vi "ME_acquire_18_DeltaForce_Daq_SteppingMode.vi"() -> ()   [LabVIEW 2015]
doc: "Use this template to build a producer/consumer design pattern. Use this template when you need to execute a process, such as data analysis, when a data source, such as a triggered acquisition, produces data at an uneven rate and you need to execute the process when the data becomes available."
uses:
  oxford_driver/Oxford Drivers/BUSGEN.LLB/OxfordAddress.ctl
  <vilib>/express/express arith-compare/Formula/XNode/ExpressFormulaBlockNode.xnode
  Mode.ctl
  <vilib>/Utility/file.llb/Write Delimited Spreadsheet (DBL).vi
  <vilib>/Analysis/NI_AALBase.lvlib
  <vilib>/Analysis/baseanly.llb/Mean (DBL).vi
  <vilib>/DAQmx/configure/timing.llb/DAQmx Timing (Sample Clock).vi
  <vilib>/DAQmx/create/channels.llb/DAQmx Create Channel (AI-Voltage-Basic).vi
  <vilib>/DAQmx/read.llb/DAQmx Read (Analog 1D DBL 1Chan NSamp).vi
panel:
  out "element":dbl
  out "TimeUp":bool
  out "meanPolarization":dbl format="%0.2f"
  out "Polarization array":dbl[](array[numeric])
  in  "First Offset?":bool
  out "Last2":dbl
  out "Actual2":dbl
  out "Up/Down":bool
  out "T array":dbl[](array[numeric])
  out "Averaged I(T)":dbl[][](array[numeric])
  in  "Averaged P(T)":dbl[][](array[numeric])
  out "remaining elements 2":T1(array[cluster])
  out "Actual mean":dbl format="%0.6f"
  in  "Averaged dt":dbl[][](array[numeric])
  in  "Averaged P(B)":dbl[][](array[numeric])
  out "LockInR":dbl
  out "deltaUaux":dbl
  out "Actual Voltage (V)":dbl caption="Actual AuxV" step=0.1
  in  "Stop":bool
  out "SaveSweep":bool=TRUE
  out "Measurement File_dn":path
  out "Measurement File_up":path
  out "Measurement File_average":path
  out "Actual Polarization":dbl
  in  "Reset IB?":bool
  in  "First?":bool
  in  "Save Period":dbl=1.0
  out "Averaged I(B)":dbl[][](array[numeric])
  out "P(uC/mm^2)":dbl[](array[numeric])
  in  "Sweep":bool
  out "Offset array":dbl[](array[numeric])
  in  "stop 2":bool
  in  "dB":dbl=0.005
  out "appended array":dbl[][](array[numeric])
  out "Actual B Field (T)":dbl
  out "Actual Temperature (K)":dbl
  out "Actual Current (pA)":dbl
  in  "Tab Control":T2(tab)
  in  "dt (K)":dbl=0.1
  in  "Max temperature (K)":dbl=20.0
  in  "Min Temperature (K)":dbl=4.5
  out "P(T)":cluster{dbl[], dbl[]}[](graph)
  out "I(T)":cluster{dbl[], dbl[]}[](graph)
  in  "Set temperature (K)":dbl=4.5
  in  "Temp Ramping Rate (K/min)":dbl=10.0
  in  "Heater Range":enum16{"Off", "Low", "Medium", "High"}(ring)
  in  "Heater On/Off":bool
  out "Setpoint Temperature (K)":dbl
  out "I(T) /Averaged/":cluster{"B array":dbl[], dbl[]}[](graph)
  out "P(T) /Averaged/":cluster{"B array":dbl[], dbl[]}[](graph)
  in  "Stabilization Time (s)":dbl
  out "I(B) 3":cluster{dbl[], dbl[]}[](graph)
  out "I(B) /Averaged/":cluster{"B array":dbl[], dbl[]}[](graph)
  out "P(B) /Averaged/":cluster{"B array":dbl[], dbl[]}[](graph)
  out "P(B)":cluster{"yi":dbl[], dbl[]}(graph)
  in  "Set Field (T)":dbl
  in  "Go to Set":bool
  in  "Sweep Rate (T/min)":dbl=2.0 format="%.6f"
  in  "Field To Zero":bool
  out "Target Field":dbl
  in  "Min Field (T)":dbl
  in  "Max Field (T)":dbl=0.15
  in  "Threshold B (T)":dbl
  in  "ReOffset":bool
  in  "Window (s)":dbl
  in  "Field Step (T)":dbl
  in  "Stepping Mode":bool
  out "Ready2Step":bool
  in  "Dwell Time (s)":dbl
  out "B(t)":dbl(graph)
  out "I(t)":dbl(graph)
  out "P(t)":dbl(graph)
  in  "Max count array":i32[](array[numeric])=[2]
  in  "Magnetic Field array (T)":dbl[](array[numeric])=[0.025, 0.05, 0.075, 0.1, 0.125, 0.15, 0.175, 0.2, 0.225, 0.25, 0.275, 0.3]
  in  "T Sweep Rate Array":dbl[](array[numeric])=[10.0, 20.0]
  in  "secs to wait":dbl=180.0
  out "Wait (s)":dbl
  in  "Directory":string
  out "Finished":bool=TRUE
  out "Step Rate":bool
  out "New":bool=TRUE
  in  "Temperature Array":dbl[](array[numeric])=[4.5, 5.0, 6.0, 7.0, 8.0, 9.0, 10.0, 11.0, 12.0]
  in  "Sweep Rate Array":dbl[](array[numeric])=[2.0, 1.0, 0.5, 0.1, 0.05, 9.0, 10.0, 11.0, 12.0]
  in  "Record ALL":bool
  in  "Max Countl":i32
  out "i":i32
  out "j":i32
  out "Step Temp":bool
  in  "FileName":string
  in  "Measure Noise":bool
  in  "Cycles":i32
  in  "maximum value":dbl=10.0 format="%0.2f"
  in  "minimum value":dbl=-10.0 format="%0.2f"
  in  "physical channels":tag="Dev1/ai1"
  out "PSD (pA/Hz^1/2) Peaks Removed":cluster{"f0":dbl, "df":dbl, "magnitude":dbl[]}(graph)
  out "PSD (pA/Hz^1/2)":cluster{"f0":dbl, "df":dbl, "magnitude":dbl[]}(graph)
  out "Current (pA) Filtered":waveform(dbl)(graph)
  out "Current (pA)":dbl[](graph)
  in  "Samples per channel":i32=1000
  in  "Rate":dbl=1000.0 format="%0.2f"
  in  "Cut-Off Frequency":dbl=100.0 caption="Lower Cut-Off"
  in  "Filter On":bool
  in  "Count":i32=60
  in  "Keithley (IV conv) averaging":i32=10
  in  "Lock_in_Amplifier":refnum<visa-resource-name>="GPIB0::5::INSTR"
  out "Dc offset":dbl
  in  "Calibrate":bool
  in  "IV converter":refnum<visa-resource-name>="GPIB0::20::INSTR"
  in  "Magnetic Field":refnum<visa-resource-name>="GPIB0::21::INSTR"
  out "Time Lag":dbl=0.0500025749206543
  in  "Lake Shore":refnum<visa-resource-name>="GPIB0::11::INSTR"
  in  "Temp Refresh (s)":dbl=0.1
  in  "Sampling rate (Hz)":dbl=10.0
  in  "Gain (V/A)":dbl=1000000000.0
  in  "Sample area (mm^2)":dbl=1.0
  out "B_V":cluster{dbl[], "Best Linear Fit":dbl[]}[](graph)=[{[-0.00769241141, -0.00768011662, -0.0029394633, 0.00271952438, 0.00937200583, 0.0154641889, 0.0217080684, 0.0281692221, 0.0344763397, 0.0407091529, 0.0473661569, 0.0541476438, 0.0611164384, 0.0676637725, 0.073937413, 0.0801511723, 0.0863882257, 0.0933787866, 0.0997676928, 0.106163316, 0.113953626, 0.118979018, 0.126030157, 0.132855724, 0.13883398, 0.14631074, 0.153030676, 0.159156864, 0.165801088, 0.17248087, 0.178555009, 0.185285367, 0.192834407, 0.198751051, 0.205413053, 0.212847389, 0.219477697, 0.225574642, 0.232225854, 0.239015189, 0.245675966, 0.252411162, 0.258453848, 0.265211852, 0.271251534, 0.277801221, 0.284008329, 0.291402813, 0.297970768, 0.304082546, 0.310761405, 0.317366634, 0.323522001, 0.330123184, 0.336841279, 0.343557963, 0.349608435, 0.356238003, 0.363590921, 0.370338319, 0.376962983], "Best Linear Fit"=[0.0, 0.0015, 0.0035, 0.0056, 0.0076, 0.0096, 0.0116, 0.0136, 0.0156, 0.0177, 0.0197, 0.0219, 0.0239, 0.0259, 0.0279, 0.0299, 0.032, 0.034, 0.036, 0.038, 0.04, 0.042, 0.0441, 0.046, 0.048, 0.05, 0.052, 0.054, 0.056, 0.058, 0.06, 0.0621, 0.0643, 0.0663, 0.0684, 0.0704, 0.0725, 0.0745, 0.0765, 0.0787, 0.0807, 0.0827, 0.0847, 0.0868, 0.0888, 0.0908, 0.0928, 0.0948, 0.0968, 0.0988, 0.1008, 0.1028, 0.1048, 0.1069, 0.1091, 0.1111, 0.1131, 0.1152, 0.1173, 0.1193, 0.1213]}, {[-0.00769241141, -0.00768011662, -0.0029394633, 0.00271952438, 0.00937200583, 0.0154641889, 0.0217080684, 0.0281692221, 0.0344763397, 0.0407091529, 0.0473661569, 0.0541476438, 0.0611164384, 0.0676637725, 0.073937413, 0.0801511723, 0.0863882257, 0.0933787866, 0.0997676928, 0.106163316, 0.113953626, 0.118979018, 0.126030157, 0.132855724, 0.13883398, 0.14631074, 0.153030676, 0.159156864, 0.165801088, 0.17248087, 0.178555009, 0.185285367, 0.192834407, 0.198751051, 0.205413053, 0.212847389, 0.219477697, 0.225574642, 0.232225854, 0.239015189, 0.245675966, 0.252411162, 0.258453848, 0.265211852, 0.271251534, 0.277801221, 0.284008329, 0.291402813, 0.297970768, 0.304082546, 0.310761405, 0.317366634, 0.323522001, 0.330123184, 0.336841279, 0.343557963, 0.349608435, 0.356238003, 0.363590921, 0.370338319, 0.376962983], "Best Linear Fit"=[0.002353460844818253, 0.002357267374965663, 0.003824997997530172, 0.005577049655813272, 0.007636692089275871, 0.009522863265806463, 0.01145600043639222, 0.013456406815525209, 0.015409122826751182, 0.01733883381400479, 0.019399876452181594, 0.021499459635718428, 0.023657034245452215, 0.025684122519169482, 0.027626473848249778, 0.02955028565017564, 0.03148130942513291, 0.03364562299316916, 0.03562366117513693, 0.037603778974812686, 0.040015698972850115, 0.04157158615356273, 0.04375465501257369, 0.04586788562152819, 0.0477187843918964, 0.050033627699098075, 0.05211415440778254, 0.05401085368533849, 0.056067939569859164, 0.05813603439385595, 0.06001661903361471, 0.06210037244704129, 0.06443759401357516, 0.0662694173922171, 0.06833200743687069, 0.07063371605572277, 0.07268649347515121, 0.0745741389696738, 0.07663338837489471, 0.07873540137051047, 0.08079761214887074, 0.08288286343195213, 0.08475371006132383, 0.08684602281837933, 0.08871593939391825, 0.09074375613756333, 0.09266550866283872, 0.09495487889775463, 0.09698835150804998, 0.09888058937557581, 0.10094839843403076, 0.10299341126621803, 0.10489914451207855, 0.10694290468187984, 0.10902286140750632, 0.11110238128028392, 0.11297563849525552, 0.11502818680688229, 0.1173046879946565, 0.11939371707962458, 0.12144474708765744]}]
  out "V_I":cluster{dbl[], "Best Linear Fit":dbl[]}[](graph)=[{[0.0, 0.012, 0.026, 0.04, 0.054, 0.068, 0.081, 0.096, 0.11, 0.124, 0.138, 0.153, 0.167, 0.18, 0.195, 0.208, 0.223, 0.236, 0.251, 0.265, 0.279, 0.292, 0.306, 0.32, 0.334, 0.348, 0.362, 0.375, 0.389, 0.403, 0.417, 0.432, 0.446, 0.46, 0.475, 0.489, 0.504, 0.517, 0.531, 0.546, 0.56, 0.574, 0.588, 0.602, 0.616, 0.63, 0.644, 0.658, 0.672, 0.685, 0.699, 0.713, 0.727, 0.742, 0.755, 0.77, 0.784, 0.799, 0.814, 0.827, 0.841], "Best Linear Fit"=[-0.00769241141, -0.00768011662, -0.0029394633, 0.00271952438, 0.00937200583, 0.0154641889, 0.0217080684, 0.0281692221, 0.0344763397, 0.0407091529, 0.0473661569, 0.0541476438, 0.0611164384, 0.0676637725, 0.073937413, 0.0801511723, 0.0863882257, 0.0933787866, 0.0997676928, 0.106163316, 0.113953626, 0.118979018, 0.126030157, 0.132855724, 0.13883398, 0.14631074, 0.153030676, 0.159156864, 0.165801088, 0.17248087, 0.178555009, 0.185285367, 0.192834407, 0.198751051, 0.205413053, 0.212847389, 0.219477697, 0.225574642, 0.232225854, 0.239015189, 0.245675966, 0.252411162, 0.258453848, 0.265211852, 0.271251534, 0.277801221, 0.284008329, 0.291402813, 0.297970768, 0.304082546, 0.310761405, 0.317366634, 0.323522001, 0.330123184, 0.336841279, 0.343557963, 0.349608435, 0.356238003, 0.363590921, 0.370338319, 0.376962983]}, {[0.0, 0.012, 0.026, 0.04, 0.054, 0.068, 0.081, 0.096, 0.11, 0.124, 0.138, 0.153, 0.167, 0.18, 0.195, 0.208, 0.223, 0.236, 0.251, 0.265, 0.279, 0.292, 0.306, 0.32, 0.334, 0.348, 0.362, 0.375, 0.389, 0.403, 0.417, 0.432, 0.446, 0.46, 0.475, 0.489, 0.504, 0.517, 0.531, 0.546, 0.56, 0.574, 0.588, 0.602, 0.616, 0.63, 0.644, 0.658, 0.672, 0.685, 0.699, 0.713, 0.727, 0.742, 0.755, 0.77, 0.784, 0.799, 0.814, 0.827, 0.841], "Best Linear Fit"=[-0.015941127780698654, -0.010342478990544012, -0.0038107220686969304, 0.0027210348531501527, 0.009252791774997235, 0.01578454869684432, 0.02184975155284518, 0.028848062540538483, 0.03537981946238557, 0.041911576384232645, 0.048443333306079736, 0.05544164429377303, 0.061973401215620116, 0.06803860407162098, 0.07503691505931429, 0.08110211791531513, 0.08810042890300844, 0.0941656317590093, 0.10116394274670261, 0.1076956996685497, 0.11422745659039678, 0.12029265944639762, 0.1268244163682447, 0.1333561732900918, 0.13988793021193888, 0.14641968713378595, 0.15295144405563305, 0.15901664691163392, 0.165548403833481, 0.1720801607553281, 0.17861191767717516, 0.18561022866486845, 0.19214198558671555, 0.19867374250856262, 0.20567205349625592, 0.212203810418103, 0.2192021214057963, 0.22526732426179719, 0.23179908118364426, 0.23879739217133758, 0.24532914909318465, 0.2518609060150317, 0.2583926629368788, 0.2649244198587259, 0.271456176780573, 0.27798793370242003, 0.28451969062426713, 0.29105144754611423, 0.2975832044679613, 0.3036484073239622, 0.31018016424580924, 0.3167119211676563, 0.3232436780895034, 0.3302419890771967, 0.3363071919331976, 0.3433055029208909, 0.34983725984273795, 0.35683557083043127, 0.36383388181812454, 0.3698990846741254, 0.3764308415959725]}]
  out "B0 (T)":dbl=0.0026443907573365636
  out "B/V (T/V)":dbl=0.3027997253900218
  out "I0 (A)":dbl=-0.008736391445912099
  out "V/I (Ohm)":dbl=0.4773805959957447
  in  "Offset?":bool
  in  "Magnet":bool=TRUE
  in  "Ramp":bool=TRUE
  in  "DaQ":bool
  in  "Moving average":i8=10
  in  "Sample Rate":dbl=1000.0
  in  "Number of Samples":i32=100
  in  "Physical Channel":tag="kartya/ai0"
  in  "Min Voltage":dbl=-5.0
  in  "Max Voltage":dbl=5.0
  in  "Terminal Configuration":i32(ring)=-1 items=["default"=-1, "RSE"=10083, "NRSE"=10078, "Differential"=10106, "Pseudodifferential"=12529]
  out "Confirm":bool
  in  "Dwell Time (ms)":u32=1000
  in  "Temp/Magnetic Field":bool
  out "index":i8
  out "Read?":bool
  out "Magnetic Field (T)":dbl[](array[numeric])
  out "Reset":bool
  out "Measured Current (pA)":dbl[](array[numeric])
  out "Elapsed Time (s)":dbl[](array[numeric])
  out "Start time":timestamp
  in  "Enum":T3=enum."Process"
  out "B array":dbl[](array[numeric])
  in  "dB (T)":dbl=0.0025
  in  "Counter":i8
  out "L magnet (H)":dbl
  out "R magnet (mOhm)":dbl
  out "Actual Current (R0)":dbl
  out "Actual Field (T)":dbl
  out "Temperature array":dbl[](array[numeric])
  in  "New Measurement File":bool
  out "Measurement File":path
  out "refnum out":refnum<file>
  in  "Measuring":bool
  in  "Measure /Pause":bool
  in  "stop":bool
  # "DeltaForce"
  # "Discrete"
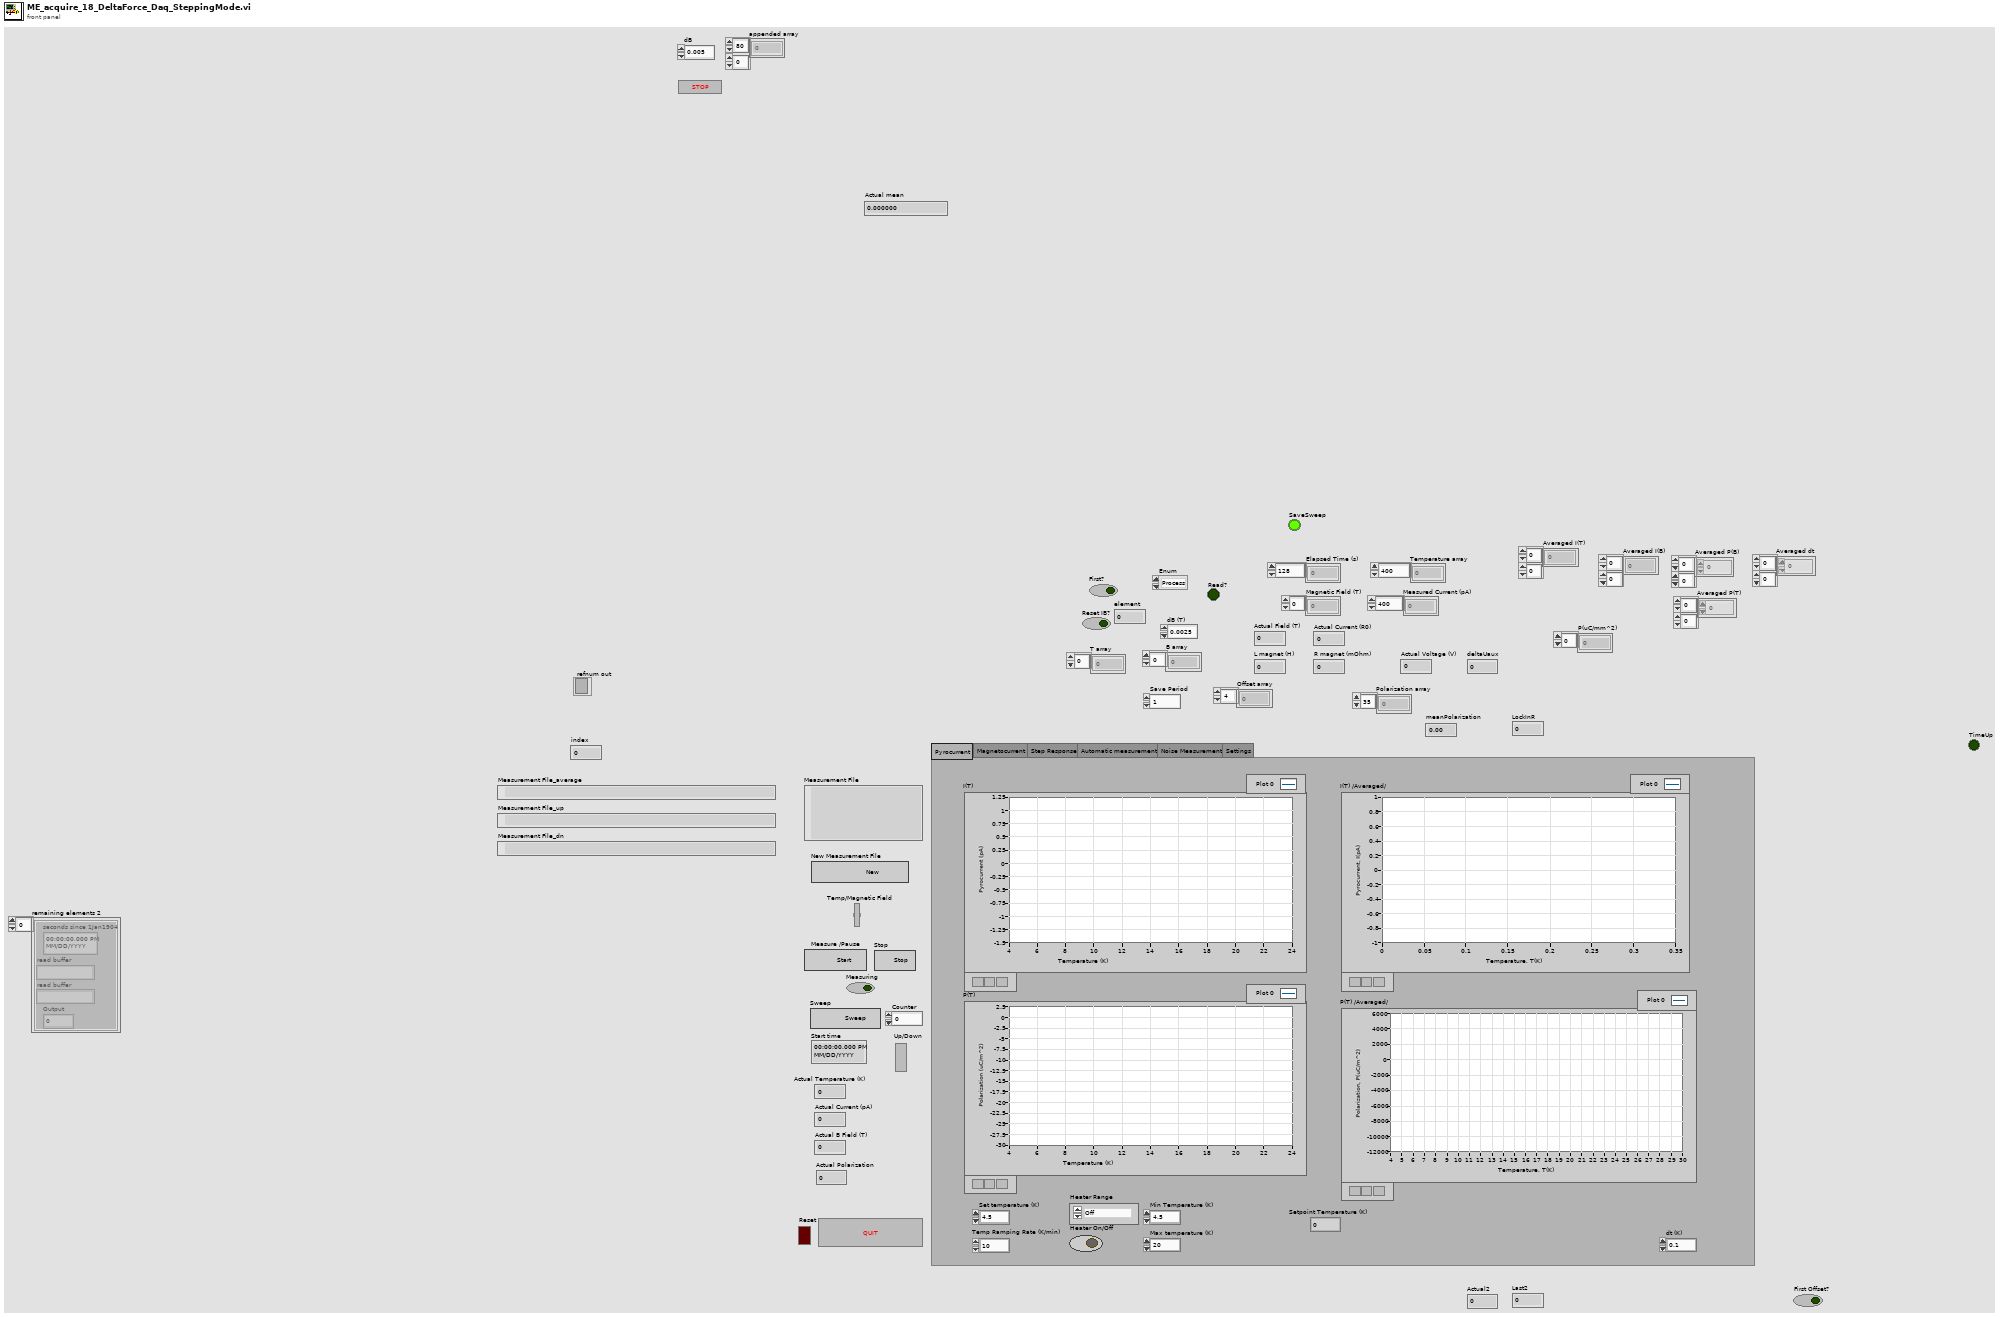
[diagram p1: front panel]
types:
  T1 = cluster{"seconds since 1Jan1904":timestamp, "read buffer":string, "read buffer":string, "Output":dbl}[]
  T2 = enum32{"Pyrocurrent", "Magnetocurrent", "Step Response", "Automatic measurement", "Noise Measurement", "Settings"}
  T3 = typedef "Mode.ctl" = enum16{"Offset", "Process", "Sweep", "StepOxford", "StepDelta", "Plot", "Save", "New", "Return", ""}
  T4 = cluster{"seconds since 1Jan1904":timestamp, "read buffer":string, "read buffer":string, "Output":dbl}
  T5 = enum16{"open", "replace", "create", "open or create", "replace or create", "replace or create with confirmation"}
  T6 = typedef "OxfordAddress.ctl" = cluster{"Com Port":i32, "ISOBUS Address":i32, "GPIB Address":i16, "Communication":enum16{"RS232", "ISOBUS", "GPIB", "Gateway"}}
  T7 = cluster{"B array":dbl[], "Averaged P(B)":dbl[]}[]
  T8 = cluster{"B array":dbl[], "Averaged P(B) Out":dbl[]}
  T9 = cluster{"B array":dbl[], "BaselineSubtracted I(B)":dbl[]}
  T10 = cluster{"B array":dbl[], "Averaged P(B) Out":dbl[]}[]
  T11 = cluster{"B array":dbl[], "BaselineSubtracted I(B)":dbl[]}[]
  T12 = cluster{"T array":dbl[], "Averaged P(T) Out":dbl[]}
  T13 = cluster{"T array":dbl[], "Averaged I(B) out":dbl[]}
  T14 = cluster{"T array":dbl[], "Averaged P(T) Out":dbl[]}[]
  T15 = cluster{"T array":dbl[], "Averaged I(B) out":dbl[]}[]
  T16 = cluster{"I array out (A)":dbl[], "V array out (V)":dbl[]}
  T17 = cluster{"I array out (A)":dbl[], "Best Linear Fit":dbl[]}
  T18 = cluster{"V array out (V)":dbl[], "B array Out":dbl[]}
  T19 = cluster{"V array out (V)":dbl[], "Best Linear Fit 2":dbl[]}
  T20 = cluster{"I array out (A)":dbl[], "Best Linear Fit":dbl[]}[]
  T21 = cluster{"V array out (V)":dbl[], "Best Linear Fit 2":dbl[]}[]
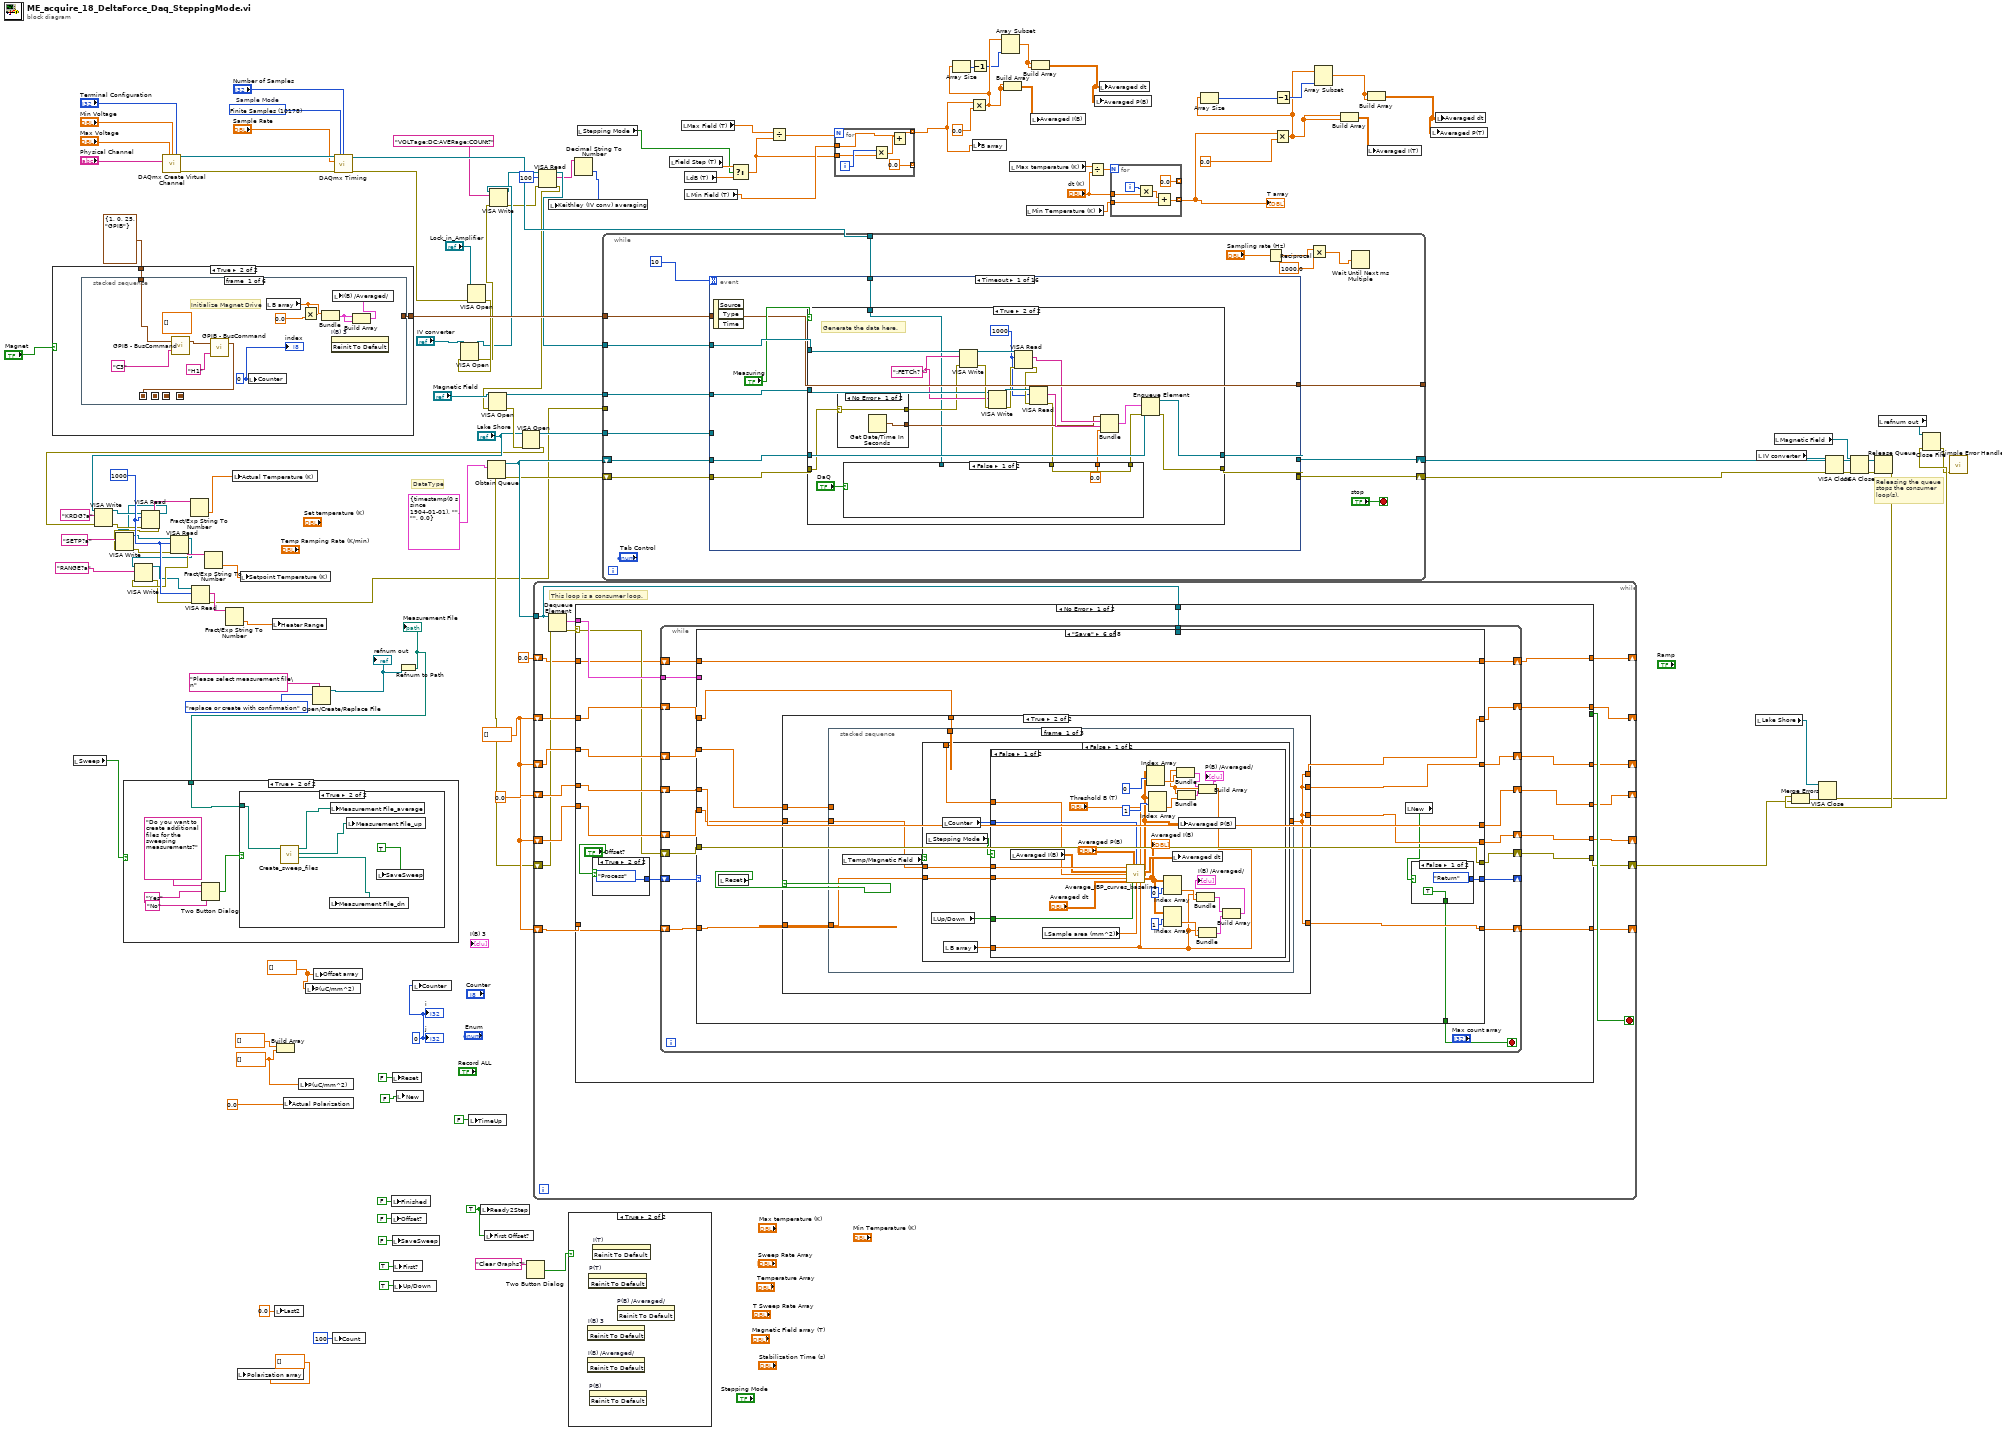
[diagram p0: block diagram]
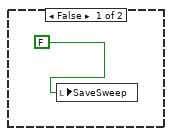
[diagram p4: hidden frame]
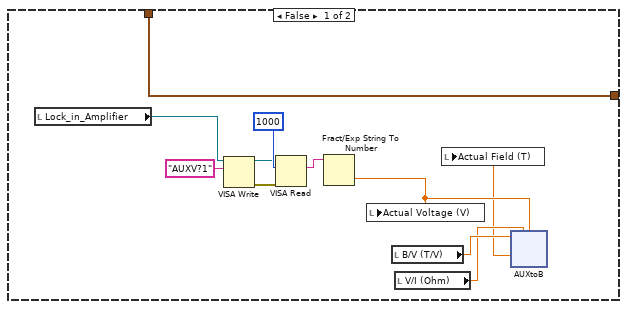
[diagram p5: hidden frame]
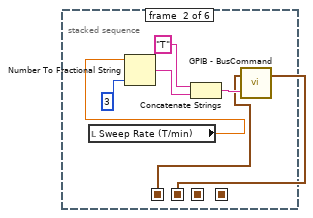
[diagram p6: hidden frame]
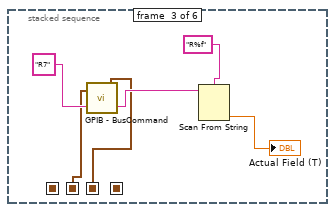
[diagram p7: hidden frame]
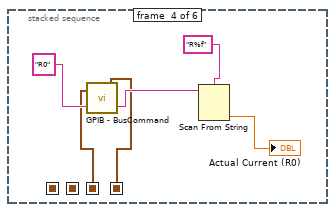
[diagram p8: hidden frame]
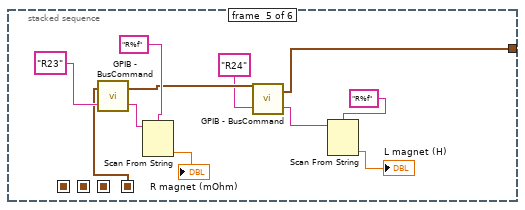
[diagram p9: hidden frame]
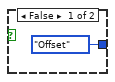
[diagram p11: hidden frame]
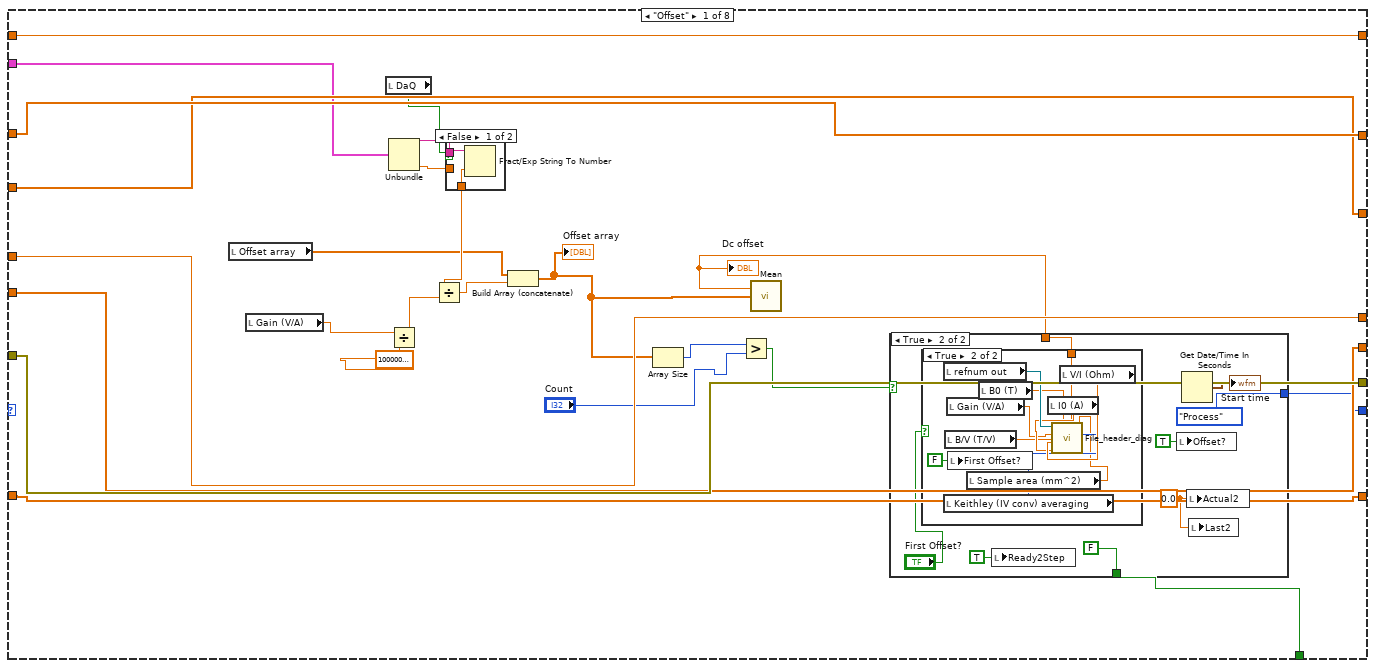
[diagram p12: hidden frame]
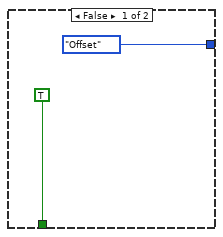
[diagram p14: hidden frame]
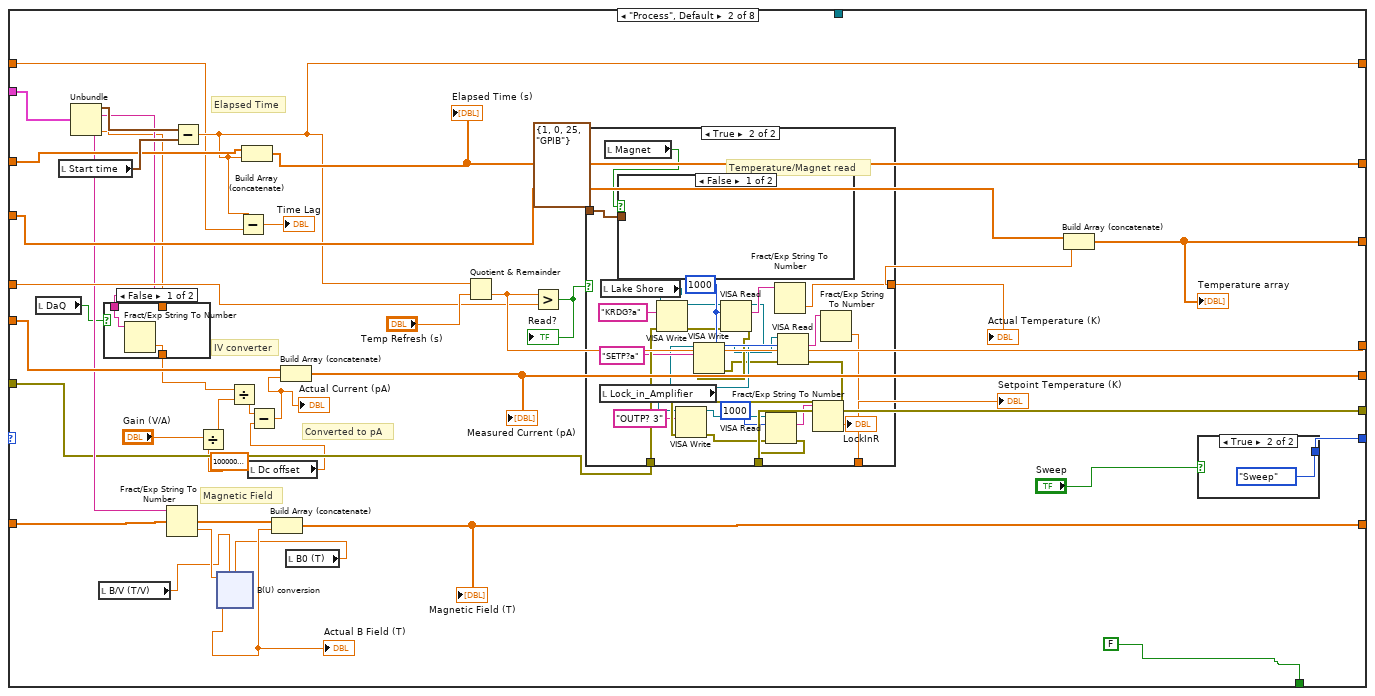
[diagram p16: hidden frame]
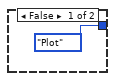
[diagram p18: hidden frame]
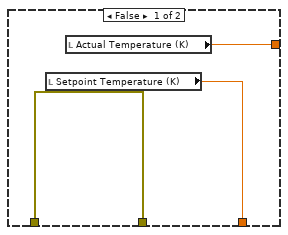
[diagram p19: hidden frame]
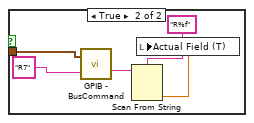
[diagram p20: hidden frame]
diagram:
  w9 = TRUE ("Ready2Step")
  w44 = 10178 items=["Finite Samples"=10178, "Continuous Samples"=10123, "Hardware Timed Single Point"=12522]  # Sample Mode
  w71 = u32 1000 ("byte count")
  w82 = 0 ("j")
  w79 = dbl[] []
  w95 = dbl[] []
  w101 = dbl[] []
  # "DataType"
  # "Releasing the queue stops the consumer loop(s)."
  n1 = case shown="True" "Magnet" {
    tunnel: T6 {"Com Port"=1, "ISOBUS Address"=0, "GPIB Address"=25, "Communication"=enum."GPIB"} ("Address") -> [w135 w149]
    tunnel: [w135 w148] -> w107
    frame False {
      n2 = local read "Lock_in_Amplifier"() -> (w129:refnum<visa-resource-name>)
      n3 = VISA Write(VISA resource name=w129, write buffer="AUXV?1") -> (VISA resource name out=w130:refnum<visa-resource-name>, error out=w134:errorcluster)  [unwired: 1 in, 1 out]
      n4 = VISA Read(VISA resource name=w130, byte count=u32 1000, error in (no error)=w134) -> (read buffer=w133:string)  [unwired: 3 out]
      n5 = Fract/Exp String To Number(string=w133) -> (number=w126:dbl)  [unwired: 3 in, 1 out]
      n6 = local write "Actual Voltage (V)"(w126) -> ()
      n7 = local read "B/V (T/V)"() -> (w128:dbl)
      n8 = local read "V/I (Ohm)"() -> (w127:dbl)
      n9 = xnode "AUXtoB"("BpV"=w128, "Rm"=w127, "Aux"=w126) -> ("Result"=w125:dbl)  [unwired: 1 in, 1 out]
      n10 = local write "Actual Field (T)"(w125) -> ()
    }
    frame True {
      n11 = stacked-sequence {
        seq-local: [w157 _ _ _ _ _] -> [_ w162 _ _ _ _]
        seq-local: [_ w161 _ _ _ _] -> [_ _ w169 _ _ _]
        seq-local: [_ _ w168 _ _ _] -> [_ _ _ w175 _ _]
        seq-local: [_ _ _ w174 _ _] -> [_ _ _ _ w186 _]
        tunnel: w149 -> [w159 _ _ _ _ _]
        tunnel: [_ _ _ _ w184 _] -> w148
        frame #0 {
          (unwired) dbl[][] []
          w155 = i8 0 ("Counter")
          # "Initialize Magnet Drive"
          n12 = call "GPIB - BusCommand.vi"("Command"="C3", "Address"=w159) -> ("Address(thru)"=w158:T6)  [unwired: 1 out]
          n13 = call "GPIB - BusCommand.vi"("Command"="H1", "Address"=w158) -> ("Address(thru)"=w157:T6)  [unwired: 1 out]
          n14 = local write "Counter"(w155) -> ()
          n15 = local read "B array"() -> (w153:dbl[])
          n16 = Multiply(x=w153, y=0.0) -> (x*y=w152:dbl[])
          n17 = Bundle("B array"=w153, w152) -> (w151:cluster{"B array":dbl[], dbl[]})  [unwired: 1 in]
          n18 = invoke on="I(B) 3" class="XYGraph (strict)" method="Reinit To Default"() -> ()  [unwired: 3 in, 3 out]
          n19 = Build Array(w151, w151) -> (w150:cluster{"B array":dbl[], dbl[]}[])
          n20 = local write "I(B) /Averaged/"(w150) -> ()
          "index" <- w155
        }
        frame #1 {
          n21 = local read "Sweep Rate (T/min)"() -> (w163:dbl)
          n22 = Number To Fractional String(number=w163, precision (6)=i16 3) -> (F-format string=w165:string)  [unwired: 2 in]
          n23 = Concatenate Strings("T" ("format string"), w165) -> (w164:string)
          n24 = call "GPIB - BusCommand.vi"("Command"=w164, "Address"=w162) -> ("Address(thru)"=w161:T6)  [unwired: 1 out]
        }
        frame #2 {
          n25 = call "GPIB - BusCommand.vi"("Command"="R7" ("format string"), "Address"=w169) -> ("Reply"=w173:string, "Address(thru)"=w168:T6)
          n26 = Scan From String(format string="R%f" ("remaining string"), input string=w173) -> (output 1=→"Actual Field (T)":dbl)  [unwired: 3 in, 3 out]
        }
        frame #3 {
          n27 = call "GPIB - BusCommand.vi"("Command"="R0" ("format string"), "Address"=w175) -> ("Reply"=w179:string, "Address(thru)"=w174:T6)
          n28 = Scan From String(format string="R%f" ("remaining string"), input string=w179) -> (output 1=→"Actual Current (R0)":dbl)  [unwired: 3 in, 3 out]
        }
        frame #4 {
          n29 = call "GPIB - BusCommand.vi"("Command"="R23" ("format string"), "Address"=w186) -> ("Reply"=w190:string, "Address(thru)"=w185:T6)
          n30 = Scan From String(format string="R%f" ("remaining string"), input string=w190) -> (output 1=→"R magnet (mOhm)":dbl)  [unwired: 3 in, 3 out]
          n31 = call "GPIB - BusCommand.vi"("Command"="R24" ("format string"), "Address"=w185) -> ("Reply"=w182:string, "Address(thru)"=w184:T6)
          n32 = Scan From String(format string="R%f" ("remaining string"), input string=w182) -> (output 1=→"L magnet (H)":dbl)  [unwired: 3 in, 3 out]
        }
        frame #5 {
        }
      }
    }
  }
  n33 = local read "Sweep"() -> (w87:bool)
  n34 = call-poly <vilib>:"DAQmx Create Virtual Channel.vi"("maximum value"="Max Voltage", "minimum value"="Min Voltage", "input terminal configuration"="Terminal Configuration", "physical channels"="Physical Channel") -> ("task out"=w42:refnum<k21>, "error out"=w43:errorcluster)  [unwired: 10 in]
  n35 = local write "Polarization array"(dbl[] [] ("Polarization array")) -> ()
  n36 = local write "Last2"(0.0 ("Last2")) -> ()
  n37 = Build Array(dbl[] [], w79) -> ()  [unwired: 1 out]
  n38 = local write "Actual Polarization"(0.0 ("Actual Polarization")) -> ()
  n39 = local write "P(uC/mm^2)"(w79) -> ()
  n40 = local write "P(uC/mm^2)"(w95) -> ()
  n41 = Open/Create/Replace File(prompt="Please select measurement file\n", operation (0:open)=T5."replace or create with confirmation") -> (refnum out=w104:refnum<file>)  [unwired: 4 in, 2 out]
  "refnum out" <- w104
  n42 = local write "Offset array"(w95) -> ()
  n43 = local write "Count"(100 ("Count")) -> ()
  n44 = call-poly <vilib>:"DAQmx Timing.vi"("task/channels in"=w42, "sample mode"=w44, "samples per channel"="Number of Samples", "rate"="Sample Rate", "error in"=w43) -> ("task out"=w34:refnum<k21>, "error out"=w35:errorcluster)  [unwired: 9 in]
  n45 = local write "Finished"(FALSE ("Finished")) -> ()
  n46 = local write "Offset?"(FALSE ("Offset?")) -> ()
  n47 = local write "Reset"(FALSE ("Reset")) -> ()
  n48 = local write "SaveSweep"(FALSE ("SaveSweep")) -> ()
  n49 = local write "First?"(TRUE ("First?")) -> ()
  n50 = local write "Up/Down"(TRUE ("Up/Down")) -> ()
  n51 = local write "New"(FALSE ("New")) -> ()
  n52 = Refnum to Path(1:w104) -> (0:w86:path)
  "Measurement File" <- w86
  n53 = case shown="True" w87 {
    tunnel: w86 -> [_ w191]
    frame False {
    }
    frame True {
      n54 = Two Button Dialog(message="Do you want to create additional files for the sweeping measurements?" ("string"), 1:"No" ("F button name (\"Cancel\")"), 2:"Yes" ("T button name (\"OK\")")) -> (T button?=w193:bool)
      n55 = case shown="True" w193 {
        tunnel: w191 -> [_ w201]
        frame False {
          n56 = local write "SaveSweep"(FALSE ("SaveSweep")) -> ()
        }
        frame True {
          n57 = call "Create_sweep_files.vi"("Measurement File"=w201) -> ("Path 3"=w198:path, "Path 2"=w199:path, "Path"=w200:path)  [unwired: 8 in]
          n58 = local write "Measurement File_dn"(w198) -> ()
          n59 = local write "Measurement File_average"(w200) -> ()
          n60 = local write "Measurement File_up"(w199) -> ()
          n61 = local write "SaveSweep"(TRUE) -> ()
        }
      }
    }
  }
  n62 = local write "Counter"(w82) -> ()
  n63 = VISA Open(error in (no error)=w35, VISA resource name="Lock_in_Amplifier") -> (error out=w54:errorcluster)  [unwired: 3 in, 1 out]
  n64 = VISA Open(error in (no error)=w54, VISA resource name="IV converter") -> (VISA resource name=w31:refnum<visa-resource-name>, error out=w32:errorcluster)  [unwired: 3 in]
  n65 = local write "TimeUp"(FALSE ("TimeUp")) -> ()
  n66 = local write "Ready2Step"(w9) -> ()
  n67 = local write "First Offset?"(w9) -> ()
  n68 = Obtain Queue(element data type=T4 {"seconds since 1Jan1904"=timestamp(0 s since 1904-01-01), "read buffer"="", "read buffer"="", "Output"=0.0} ("output cluster")) -> (queue out=w124:refnum<queue>, error out=w99:errorcluster)  [unwired: 4 in, 1 out]
  n69 = VISA Write(VISA resource name=w31, write buffer="VOLTage:DC:AVERage:COUNt?", error in (no error)=w32) -> (VISA resource name out=w27:refnum<visa-resource-name>, error out=w29:errorcluster)  [unwired: 1 out]
  n70 = Two Button Dialog(message="Clear Graphs?") -> (T button?=w81:bool)  [unwired: 2 in]
  n71 = while {
    tunnel: w124 -> [w202]
    shift-right: [w215] -> _
    shift-left: w101 -> [w214]
    shift-right: [w213] -> _
    shift-left: w101 -> [w212]
    shift-right: [w211] -> _
    shift-left: w101 -> [w210]
    shift-right: [w209] -> _
    shift-left: 0.0 -> [w208]
    shift-right: [w207] -> _
    shift-left: w101 -> [w206]
    shift-right: [w216] -> w112
    shift-left: w99 -> [w205]
    shift-right: [w204] -> _
    shift-left: 0.0 -> [w203]
    stop <- w217 stop-if-true
    # "This loop is a consumer loop."
    n72 = Dequeue Element(queue=w202, error in (no error)=w205) -> (element=w218:T4, error out=w219:errorcluster)  [unwired: 1 in, 2 out]
    n73 = case shown="No Error" w219 {
      selector: w219 -> [w225 w1176]
      tunnel: w218 -> [w236 _]
      tunnel: [_ TRUE] -> w217
      tunnel: [w224 w1176] -> w216
      tunnel: [w235 w1175] -> w215
      tunnel: w214 -> [w234 w1175]
      tunnel: [w233 w1172] -> w213
      tunnel: w212 -> [w232 w1172]
      tunnel: [w231 w1171] -> w211
      tunnel: w210 -> [w230 w1171]
      tunnel: [w229 w1173] -> w209
      tunnel: w208 -> [w228 w1173]
      tunnel: [w227 w1174] -> w207
      tunnel: w206 -> [w226 w1174]
      tunnel: [w223 w1170] -> w204
      tunnel: w203 -> [w222 w1170]
      tunnel: w202 -> [w220 _]
      frame No Error {
        n74 = case shown="True" "Offset?" {
          tunnel: [Mode."Offset" ("Enum") Mode."Process" ("Enum")] -> w237
          frame False {
          }
          frame True {
          }
        }
        n75 = while {
          shift-right: [w246] -> _
          shift-left: w237 -> [w258]
          tunnel: w236 -> [w257]
          shift-right: [w256] -> w235
          shift-left: w234 -> [w255]
          shift-right: [w248] -> w227
          shift-left: w226 -> [w247]
          shift-right: [w250] -> w229
          shift-left: w228 -> [w249]
          shift-right: [w254] -> w233
          shift-left: w232 -> [w253]
          shift-right: [w244] -> w224
          shift-left: w225 -> [w245]
          shift-right: [w252] -> w231
          shift-left: w230 -> [w251]
          shift-right: [w242] -> w223
          shift-left: w222 -> [w241]
          tunnel: w220 -> [w240]
          stop <- w243 stop-if-true
          n76 = case shown="\"Save\"" w258 {
            selector: w258 -> [_ _ _ _ _ _ _ w1163]
            tunnel: w257 -> [w276 w344 _ _ _ _ _ _]
            tunnel: [w282 w341 w402 w549 w702 w821 w939 w1168] -> w256
            tunnel: w255 -> [w282 w334 w402 w549 w702 w817 w939 w1168]
            tunnel: [w277 w340 w405 w546 w704 w823 w937 w1165] -> w254
            tunnel: w253 -> [w277 w339 w405 w546 w704 w818 w937 w1165]
            tunnel: [w278 w338 w407 w545 w699 w824 w935 w1162] -> w252
            tunnel: w251 -> [w278 w337 w407 w545 w699 w819 w935 w1162]
            tunnel: [w280 w333 w404 w547 w700 w827 0.0 w1166] -> w250
            tunnel: w249 -> [w280 w332 w404 w547 w700 w827 _ w1166]
            tunnel: [w281 w329 w403 w548 w701 w822 w938 w1167] -> w248
            tunnel: w247 -> [w281 w330 w403 w548 w701 w820 w938 w1167]
            tunnel: [w266 w327 w400 w539 Mode."Save" ("Enum") w828 Mode."Return" ("Enum") w1163] -> w246
            tunnel: w245 -> [w279 w325 w409 w543 w707 w826 w931 w1164]
            tunnel: [w279 w324 w408 w542 w707 w826 w930 w1164] -> w244
            tunnel: [w262 FALSE FALSE FALSE FALSE w815 TRUE TRUE] -> w243
            tunnel: [w265 w321 w401 w540 w703 w825 0.0 w1169] -> w242
            tunnel: w241 -> [w265 w320 w401 w540 w703 w825 _ w1169]
            tunnel: w240 -> [_ _ _ _ _ _ w929 _]
            frame "Offset" {
              n77 = local read "Offset array"() -> (w270:dbl[])
              n78 = local read "Gain (V/A)"() -> (w274:dbl)
              n79 = local read "DaQ"() -> (w261:bool)
              n80 = Unbundle(w276) -> ("read buffer"=w264:string, "Output"=w260:dbl)  [unwired: 2 out]
              n81 = Divide(x=w274, y=1000000000000.0) -> (x/y=w272:dbl)
              n82 = case shown="False" w261 {
                tunnel: [w284 w285] -> w275
                tunnel: w264 -> [w283 _]
                tunnel: w260 -> [_ w285]
                frame False {
                  n83 = Fract/Exp String To Number(string=w283) -> (number=w284:dbl)  [unwired: 3 in, 1 out]
                }
                frame True {
                }
              }
              n84 = Divide(x=w275, y=w272) -> (x/y=w271:dbl)
              n85 = Build Array (concatenate)(w270, w271) -> (w267:dbl[])
              "Offset array" <- w267
              n86 = Array Size(array=w267) -> (size(s)=w269:i32)
              n87 = Greater?(x=w269, y="Count") -> (0:w268:bool)
              n88 = call-poly <vilib>:"Mean.vi"("X"=w267) -> ("mean"=w263:dbl)  [unwired: 1 out]
              "Dc offset" <- w263
              n89 = case shown="True" w268 {
                tunnel: [Mode."Offset" ("Enum") Mode."Process" ("Enum")] -> w266
                tunnel: w263 -> [_ w293]
                tunnel: [TRUE FALSE] -> w262
                frame False {
                }
                frame True {
                  w289 = 0.0 ("Actual2")
                  n90 = case shown="True" "First Offset?" {
                    tunnel: w293 -> [_ w299]
                    frame False {
                    }
                    frame True {
                      n91 = local read "refnum out"() -> (w305:refnum<file>)
                      n92 = local read "Keithley (IV conv) averaging"() -> (w298:i32)
                      n93 = local read "B/V (T/V)"() -> (w300:dbl)
                      n94 = local read "Gain (V/A)"() -> (w301:dbl)
                      n95 = local write "First Offset?"(FALSE ("First Offset?")) -> ()
                      n96 = local read "Sample area (mm^2)"() -> (w297:dbl)
                      n97 = local read "B0 (T)"() -> (w302:dbl)
                      n98 = local read "I0 (A)"() -> (w303:dbl)
                      n99 = local read "V/I (Ohm)"() -> (w304:dbl)
                      n100 = call "File_header_diag.vi"("Averaging"=w298, "Sample area"=w297, "OFFSET"=w299, "B0"=w302, "B/V"=w300, "I0"=w303, "V/I"=w304, "Gain"=w301, "Byte Stream File in"=w305) -> ()  [unwired: 3 in]
                    }
                  }
                  n101 = local write "Ready2Step"(TRUE ("Ready2Step")) -> ()
                  n102 = local write "Offset?"(TRUE ("Offset?")) -> ()
                  n103 = Get Date/Time In Seconds() -> (seconds since 1Jan1904=→"Start time":timestamp)
                  n104 = local write "Actual2"(w289) -> ()
                  n105 = local write "Last2"(w289) -> ()
                }
              }
            }
            frame "Process", Default {
              # "Converted to pA"
              # "Magnetic Field"
              # "IV converter"
              # "Elapsed Time"
              n106 = local read "DaQ"() -> (w308:bool)
              n107 = local read "Start time"() -> (w342:timestamp)
              n108 = Unbundle(w344) -> ("seconds since 1Jan1904"=w343:timestamp, "read buffer"=w309:string, "read buffer"=w326:string, "Output"=w306:dbl)
              n109 = local read "B/V (T/V)"() -> (w316:dbl)
              n110 = case shown="False" w308 {
                tunnel: w309 -> [w348 _]
                tunnel: [w347 w349] -> w307
                tunnel: w306 -> [_ w349]
                frame False {
                  n111 = Fract/Exp String To Number(string=w348) -> (number=w347:dbl)  [unwired: 3 in, 1 out]
                }
                frame True {
                }
              }
              n112 = Fract/Exp String To Number(string=w326) -> (number=w336:dbl)  [unwired: 3 in, 1 out]
              n113 = Subtract(x=w343, y=w342) -> (x-y=w321:dbl)
              n114 = Divide(x="Gain (V/A)", y=1000000000000.0) -> (x/y=w319:dbl)
              n115 = Divide(x=w307, y=w319) -> (x/y=w314:dbl)
              n116 = Subtract(x=w321, y=w320) -> (x-y=→"Time Lag":dbl)
              n117 = Build Array (concatenate)(w334, w321) -> (w341:dbl[])
              "Elapsed Time (s)" <- w341
              n118 = local read "Dc offset"() -> (w312:dbl)
              n119 = Subtract(x=w314, y=w312) -> (x-y=w313:dbl)
              "Actual Current (pA)" <- w313
              n120 = Build Array (concatenate)(w339, w313) -> (w340:dbl[])
              "Measured Current (pA)" <- w340
              n121 = local read "B0 (T)"() -> (w315:dbl)
              n122 = xnode "B(U) conversion"("V"=w336, "BpV"=w316, "B0"=w315) -> ("Result"=w335:dbl)  [unwired: 1 in, 1 out]
              "Actual B Field (T)" <- w335
              n123 = Build Array (concatenate)(w337, w335) -> (w338:dbl[])
              "Magnetic Field (T)" <- w338
              n124 = Quotient & Remainder(x=w321, y="Temp Refresh (s)") -> (floor(x/y)=w333:dbl)  [unwired: 1 out]
              n125 = Greater?(x=w333, y=w332) -> (0:w331:bool)
              "Read?" <- w331
              n126 = case shown="True" w331 {
                tunnel: [w353 w378] -> w328
                tunnel: w325 -> [w354 w377]
                tunnel: [w354 w357] -> w324
                tunnel: T6 {"Com Port"=1, "ISOBUS Address"=0, "GPIB Address"=25, "Communication"=enum."GPIB"} ("Address") -> [_ w376]
                tunnel: [w352 w372] -> w310
                frame False {
                  n127 = local read "Setpoint Temperature (K)"() -> (w352:dbl)
                  n128 = local read "Actual Temperature (K)"() -> (w353:dbl)
                }
                frame True {
                  w373 = u32 1000 ("byte count")
                  # "Temperature/Magnet read"
                  n129 = local read "Lock_in_Amplifier"() -> (w361:refnum<visa-resource-name>)
                  n130 = local read "Lake Shore"() -> (w375:refnum<visa-resource-name>)
                  n131 = local read "Magnet"() -> (w364:bool)
                  n132 = case shown="False" w364 {
                    tunnel: w376 -> [_ w382]
                    frame False {
                    }
                    frame True {
                      n133 = call "GPIB - BusCommand.vi"("Command"="R7" ("format string"), "Address"=w382) -> ("Reply"=w383:string)  [unwired: 1 out]
                      n134 = Scan From String(format string="R%f" ("remaining string"), input string=w383) -> (output 1=w381:dbl)  [unwired: 3 in, 3 out]
                      n135 = local write "Actual Field (T)"(w381) -> ()
                    }
                  }
                  n136 = VISA Write(VISA resource name=w375, write buffer="KRDG?a", error in (no error)=w377) -> (VISA resource name out=w371:refnum<visa-resource-name>, error out=w369:errorcluster)  [unwired: 1 out]
                  n137 = VISA Read(VISA resource name=w371, byte count=w373, error in (no error)=w369) -> (VISA resource name out=w370:refnum<visa-resource-name>, read buffer=w379:string, error out=w368:errorcluster)  [unwired: 1 out]
                  n138 = VISA Write(VISA resource name=w370, write buffer="SETP?a", error in (no error)=w368) -> (VISA resource name out=w366:refnum<visa-resource-name>, error out=w367:errorcluster)  [unwired: 1 out]
                  n139 = Fract/Exp String To Number(string=w379) -> (number=w378:dbl)  [unwired: 3 in, 1 out]
                  n140 = VISA Read(VISA resource name=w366, byte count=w373, error in (no error)=w367) -> (read buffer=w365:string, error out=w363:errorcluster)  [unwired: 2 out]
                  n141 = VISA Write(VISA resource name=w361, write buffer="OUTP? 3", error in (no error)=w363) -> (VISA resource name out=w360:refnum<visa-resource-name>, error out=w362:errorcluster)  [unwired: 1 out]
                  n142 = VISA Read(VISA resource name=w360, byte count=u32 1000, error in (no error)=w362) -> (read buffer=w356:string, error out=w357:errorcluster)  [unwired: 2 out]
                  n143 = Fract/Exp String To Number(string=w356) -> (number=→"LockInR":dbl)  [unwired: 3 in, 1 out]
                  n144 = Fract/Exp String To Number(string=w365) -> (number=w372:dbl)  [unwired: 3 in, 1 out]
                }
              }
              "Actual Temperature (K)" <- w328
              "Setpoint Temperature (K)" <- w310
              n145 = Build Array (concatenate)(w330, w328) -> (w329:dbl[])
              "Temperature array" <- w329
              n146 = case shown="True" "Sweep" {
                tunnel: [Mode."Plot" ("Enum") Mode."Sweep" ("Enum")] -> w327
                frame False {
                }
                frame True {
                }
              }
            }
            frame "Sweep" {
              n147 = local read "Temp/Magnetic Field"() -> (w399:bool)
              n148 = case shown="False" w399 {
                tunnel: w409 -> [w422 w487]
                tunnel: [w421 w486] -> w408
                frame False {
                  n149 = local read "Stepping Mode"() -> (w416:bool)
                  n150 = local read "Actual Field (T)"() -> (w418:dbl)
                  n151 = local read "Min Field (T)"() -> (w417:dbl)
                  n152 = case shown="True" w416 {
                    tunnel: [w424 w425] -> w415
                    frame False {
                      n153 = local read "Read?"() -> (w424:bool)
                    }
                    frame True {
                      n154 = local read "Ready2Step"() -> (w425:bool)
                    }
                  }
                  n155 = local read "Max Field (T)"() -> (w423:dbl)
                  n156 = Greater Or Equal?(x=w417, y=w418) -> (x >= y?=w420:bool)
                  n157 = Compound Arithmetic op=AND(w420, w415) -> (w419:bool)
                  n158 = case shown="False" w419 {
                    tunnel: [w428 w467] -> w421
                    tunnel: w423 -> [w426 w466]
                    tunnel: w417 -> [_ w465]
                    tunnel: w418 -> [_ w463]
                    tunnel: w422 -> [w429 w462]
                    frame True {
                      # "Ramp Up"
                      n159 = case shown="False" "First?" {
                        tunnel: [TRUE ("Save") FALSE ("Save")] -> w432
                        tunnel: [w454 w458] -> w431
                        frame False {
                          n160 = local read "Counter"() -> (w457:i8)
                          n161 = local write "Actual Polarization"(0.0 ("Actual Polarization")) -> ()
                          n162 = Increment(x=w457) -> (x+1=w454:i8)
                          n163 = local write "Counter"(w454) -> ()
                        }
                        frame True {
                          n164 = local read "Counter"() -> (w458:i8)
                          n165 = local write "First?"(FALSE ("First?")) -> ()
                        }
                      }
                      "Reset" <- w432
                      n166 = local write "Read?"(FALSE ("Read?")) -> ()
                      n167 = local read "Record ALL"() -> (w427:bool)
                      n168 = case shown="False" w427 {
                        tunnel: w431 -> [_ w439]
                        tunnel: [FALSE w437] -> w430
                        frame False {
                        }
                        frame True {
                          n169 = Greater?(x=w439, y="Max Countl") -> (0:w437:bool)
                        }
                      }
                      n170 = case shown="False" w430 {
                        tunnel: w429 -> [w446 w453]
                        tunnel: [w445 w453] -> w428
                        tunnel: w426 -> [w444 _]
                        frame False {
                          n171 = local read "Stepping Mode"() -> (w442:bool)
                          n172 = local read "Magnet"() -> (w443:bool)
                          n173 = Not(x=w442) -> (.not. x?=w441:bool)
                          n174 = And(x=w441, y=w443) -> (x .and. y?=w440:bool)
                          n175 = case shown="False" w440 {
                            tunnel: w446 -> [w447 w450]
                            tunnel: [w447 w449] -> w445
                            tunnel: w444 -> [_ w448]
                            frame False {
                            }
                            frame True {
                              n176 = call "Set_B.vi"("error in (no error)"=w450, "address string"="25", "Set Field (T)"=w448) -> ("error out"=w449:errorcluster)  [unwired: 8 in]
                            }
                          }
                          "Target Field" <- w444
                        }
                        frame True {
                          "New" <- TRUE
                        }
                      }
                      "Up/Down" <- FALSE ("Up/Down")
                    }
                    frame False {
                      n177 = Less Or Equal?(x=w466, y=w463) -> (x <= y?=w464:bool)
                      n178 = case shown="False" w464 {
                        tunnel: [w468 w475] -> w467
                        tunnel: w465 -> [_ w473]
                        tunnel: w462 -> [w468 w476]
                        frame False {
                        }
                        frame True {
                          # "Resetting at the end of every cycle"
                          # "Ramp Dn"
                          n179 = local write "Up/Down"(TRUE ("Up/Down")) -> ()
                          n180 = local read "Stepping Mode"() -> (w472:bool)
                          n181 = local read "Magnet"() -> (w470:bool)
                          n182 = local write "Target Field"(w473) -> ()
                          n183 = Not(x=w472) -> (.not. x?=w471:bool)
                          n184 = And(x=w470, y=w471) -> (x .and. y?=w469:bool)
                          n185 = local write "Reset"(TRUE ("Reset")) -> ()
                          n186 = case shown="True" w469 {
                            tunnel: w476 -> [w478 w481]
                            tunnel: [w478 w480] -> w475
                            tunnel: w473 -> [_ w479]
                            frame False {
                            }
                            frame True {
                              n187 = call "Set_B.vi"("error in (no error)"=w481, "address string"="25", "Set Field (T)"=w479) -> ("error out"=w480:errorcluster)  [unwired: 8 in]
                            }
                          }
                        }
                      }
                      n188 = local write "Read?"(FALSE ("Read?")) -> ()
                    }
                  }
                }
                frame True {
                  n189 = local read "Setpoint Temperature (K)"() -> (w485:dbl)
                  n190 = local read "Min Temperature (K)"() -> (w484:dbl)
                  n191 = local read "Read?"() -> (w490:bool)
                  n192 = local read "Max temperature (K)"() -> (w483:dbl)
                  n193 = Equal?(x=w485, y=w484) -> (x = y?=w488:bool)
                  n194 = And(x=w488, y=w490) -> (x .and. y?=w489:bool)
                  n195 = case shown="False" w489 {
                    tunnel: [w492 w528] -> w486
                    tunnel: w483 -> [w499 w527]
                    tunnel: w484 -> [_ w526]
                    tunnel: w485 -> [_ w524]
                    tunnel: w487 -> [w493 w523]
                    frame True {
                      # "Ramp Up"
                      n196 = local read "First?"() -> (w503:bool)
                      n197 = case shown="False" w503 {
                        tunnel: [TRUE ("Save") FALSE ("Save")] -> w495
                        tunnel: [w515 w521] -> w497
                        frame False {
                          n198 = local read "Counter"() -> (w518:i8)
                          n199 = local write "Actual Polarization"(0.0 ("Actual Polarization")) -> ()
                          n200 = Increment(x=w518) -> (x+1=w515:i8)
                          n201 = local write "Counter"(w515) -> ()
                        }
                        frame True {
                          n202 = local read "Counter"() -> (w521:i8)
                          n203 = local write "First?"(FALSE ("First?")) -> ()
                        }
                      }
                      n204 = local write "Read?"(FALSE ("Read?")) -> ()
                      n205 = local write "Up/Down"(FALSE ("Up/Down")) -> ()
                      n206 = Number To Fractional String(number=w499, precision (6)=i16 3) -> (F-format string=w501:string)  [unwired: 2 in]
                      n207 = local read "Record ALL"() -> (w498:bool)
                      n208 = Concatenate Strings("SETP 1," ("write buffer"), w501) -> (w494:string)
                      n209 = case shown="True" w498 {
                        tunnel: w497 -> [_ w514]
                        tunnel: [FALSE w513] -> w496
                        frame False {
                        }
                        frame True {
                          n210 = local read "Max Countl"() -> (w512:i32)
                          n211 = Greater?(x=w514, y=w512) -> (0:w513:bool)
                        }
                      }
                      n212 = local write "Reset"(w495) -> ()
                      n213 = case shown="True" w496 {
                        tunnel: w494 -> [w508 _]
                        tunnel: w493 -> [w506 w509]
                        tunnel: [w505 w509] -> w492
                        frame False {
                          n214 = local read "Lake Shore"() -> (w507:refnum<visa-resource-name>)
                          n215 = VISA Write(VISA resource name=w507, write buffer=w508, error in (no error)=w506) -> (error out=w505:errorcluster)  [unwired: 2 out]
                        }
                        frame True {
                          n216 = local write "New"(TRUE ("New")) -> ()
                        }
                      }
                    }
                    frame False {
                      n217 = Equal?(x=w527, y=w524) -> (x = y?=w525:bool)
                      n218 = case shown="True" w525 {
                        tunnel: [w529 w533] -> w528
                        tunnel: w526 -> [_ w532]
                        tunnel: w523 -> [w529 w534]
                        frame False {
                        }
                        frame True {
                          w530 = TRUE ("Reset")
                          # "Ramp Dn"
                          n219 = Number To Fractional String(number=w532, precision (6)=i16 3) -> (F-format string=w536:string)  [unwired: 2 in]
                          n220 = local write "Reset"(w530) -> ()
                          n221 = local write "Up/Down"(w530) -> ()
                          n222 = local read "Lake Shore"() -> (w531:refnum<visa-resource-name>)
                          n223 = Concatenate Strings("SETP 1," ("write buffer"), w536) -> (w538:string)
                          n224 = VISA Write(VISA resource name=w531, write buffer=w538, error in (no error)=w534) -> (error out=w533:errorcluster)  [unwired: 2 out]
                        }
                      }
                      n225 = local write "Read?"(FALSE ("Read?")) -> ()
                    }
                  }
                }
              }
              n226 = local read "Magnet"() -> (w398:bool)
              n227 = case shown="True" w398 {
                tunnel: [Mode."StepDelta" ("Enum") w412] -> w400
                frame False {
                }
                frame True {
                  n228 = local read "Stepping Mode"() -> (w411:bool)
                  n229 = case shown="False" w411 {
                    tunnel: [Mode."Plot" ("Enum") Mode."StepDelta" ("Enum")] -> w412
                    frame False {
                    }
                    frame True {
                    }
                  }
                }
              }
            }
            frame "StepDelta" {
              n230 = local read "Stepping Mode"() -> (w541:bool)
              n231 = case shown="True" w541 {
                tunnel: w543 -> [w552 w607]
                tunnel: [w551 w604] -> w542
                tunnel: w540 -> [_ w606]
                tunnel: [w550 w605] -> w539
                frame False {
                  n232 = flat-sequence {
                    tunnel: w552 -> [w561]
                    tunnel: [w560] -> w551
                    tunnel: [Mode."Plot" ("Enum")] -> w550
                    frame #0 {
                      # "Check if it is time to step Field"
                      n233 = local read "Sweep Rate (T/min)"() -> (w562:dbl)
                      n234 = local read "B/V (T/V)"() -> (w554:dbl)
                      n235 = local read "Time Lag"() -> (w558:dbl)
                      n236 = xnode "Sweep Delay"("SweepRate"=w562, "Resolution"=0.001 ("Voltage Step (V)"), "BpV"=w554) -> ("Result"=w559:dbl)  [unwired: 1 in, 1 out]
                      n237 = Divide(x=w558, y=w559) -> (x/y=w556:dbl)
                      n238 = Multiply(x=0.001 ("y"), y=w556) -> (x*y=w555:dbl)
                      "deltaUaux" <- w555
                      n239 = stacked-sequence {
                        tunnel: w561 -> [_ w586]
                        tunnel: [_ w585] -> w560
                        tunnel: w555 -> [w564 _]
                        frame #0 {
                          n240 = local read "Actual Voltage (V)"() -> (w569:dbl)
                          n241 = local read "Up/Down"() -> (w570:bool)
                          n242 = Add(x=w569, y=w564) -> (x+y=w566:dbl)
                          n243 = Subtract(x=w569, y=w564) -> (x-y=w565:dbl)
                          n244 = Select(t=w565, s=w570, f=w566) -> (s? t:f=w568:dbl)
                          "Actual Voltage (V)" <- w568
                          n245 = local read "V/I (Ohm)"() -> (w571:dbl)
                          n246 = local read "B/V (T/V)"() -> (w572:dbl)
                          n247 = xnode "AUXtoB"("BpV"=w572, "Rm"=w571, "Aux"=w568) -> ("Result"=w567:dbl)  [unwired: 1 in, 1 out]
                          n248 = local write "Actual Field (T)"(w567) -> ()
                        }
                        frame #1 {
                          n249 = local read "Actual Voltage (V)"() -> (w591:dbl)
                          n250 = local read "Lock_in_Amplifier"() -> (w587:refnum<visa-resource-name>)
                          n251 = Format Into String(w591) -> (resulting string=w590:string)  [unwired: 3 in, 1 out]
                          n252 = Concatenate Strings("AUXV 1,", w590) -> (w588:string)
                          n253 = VISA Write(VISA resource name=w587, write buffer=w588, error in (no error)=w586) -> (error out=w585:errorcluster)  [unwired: 2 out]
                        }
                      }
                    }
                  }
                }
                frame True {
                  n254 = local read "Up/Down"() -> (w608:bool)
                  n255 = local read "Actual Field (T)"() -> (w609:dbl)
                  n256 = stacked-sequence {
                    tunnel: "Field Step (T)" -> [w615 _ _]
                    tunnel: w609 -> [w614 _ _]
                    tunnel: w608 -> [w613 _ w658]
                    tunnel: w607 -> [w612 w631 _]
                    tunnel: [_ w629 _] -> _
                    tunnel: w606 -> [_ w629 _]
                    tunnel: [_ w632 _] -> w605
                    tunnel: [_ w631 _] -> w604
                    frame #0 {
                      n257 = local read "Ready2Step"() -> (w611:bool)
                      n258 = case shown="True" w611 {
                        tunnel: w615 -> [_ w621]
                        tunnel: w614 -> [_ w622]
                        tunnel: w613 -> [_ w620]
                        tunnel: w612 -> [w616 w619]
                        tunnel: [w616 w618] -> _
                        frame False {
                        }
                        frame True {
                          n259 = Add(x=w622, y=w621) -> (x+y=w624:dbl)
                          n260 = Subtract(x=w622, y=w621) -> (x-y=w623:dbl)
                          n261 = Select(t=w623, s=w620, f=w624) -> (s? t:f=w626:dbl)
                          n262 = call "Set_B.vi"("error in (no error)"=w619, "address string"="25", "Set Field (T)"=w626) -> ("error out"=w618:errorcluster)  [unwired: 8 in]
                          n263 = local write "Ready2Step"(FALSE ("Ready2Step")) -> ()
                        }
                      }
                    }
                    frame #1 {
                      n264 = local read "Stabilization Time (s)"() -> (w628:dbl)
                      n265 = local read "Last2"() -> (w634:dbl)
                      n266 = Quotient & Remainder(x=w629, y="Window (s)") -> (floor(x/y)=w630:dbl)  [unwired: 1 out]
                      "Actual2" <- w630
                      n267 = Greater?(x=w629, y=w628) -> (0:w627:bool)
                      n268 = Greater?(x=w630, y=w634) -> (0:w633:bool)
                      n269 = case shown="True" w633 {
                        tunnel: w630 -> [_ w647]
                        tunnel: [Mode."Plot" ("Enum") w645] -> w632
                        tunnel: w627 -> [w636 _]
                        frame False {
                          n270 = local read "Actual Current (pA)"() -> (→"I(t)":dbl)
                          n271 = local read "Actual B Field (T)"() -> (→"B(t)":dbl)
                          n272 = local read "Actual Polarization"() -> (w637:dbl)
                          "P(t)" <- w637
                          n273 = case shown="True" w636 {
                            tunnel: w637 -> [_ w641]
                            frame False {
                            }
                            frame True {
                              n274 = local read "Polarization array"() -> (w642:dbl[])
                              n275 = Build Array (concatenate)(w642, w641) -> (→"Polarization array":dbl[])
                            }
                          }
                        }
                        frame True {
                          n276 = case shown="True" "ReOffset" {
                            tunnel: [Mode."Plot" ("Enum") Mode."Offset" ("Enum")] -> w645
                            frame False {
                              "Ready2Step" <- TRUE ("Ready2Step 2")
                            }
                            frame True {
                              n277 = local read "Sampling rate (Hz)"() -> (w651:dbl)
                              n278 = local write "Offset array"(dbl[] []) -> ()
                              n279 = local write "Offset?"(FALSE ("Offset?")) -> ()
                              n280 = Reciprocal(x=w651) -> (1/x=w650:dbl)
                              n281 = Divide(x="Dwell Time (s)", y=w650) -> (x/y=w654:dbl)
                              n282 = local write "Count"(w654) -> ()
                            }
                          }
                          "Last2" <- w647
                          "TimeUp" <- TRUE ("TimeUp")
                        }
                      }
                    }
                    frame #2 {
                      n283 = local read "TimeUp"() -> (w657:bool)
                      n284 = case shown="True" w657 {
                        tunnel: w658 -> [_ w659]
                        frame False {
                        }
                        frame True {
                          n285 = stacked-sequence {
                            tunnel: w659 -> [w673 _]
                            frame #0 {
                              (unwired) 1 ("index")
                              n286 = local read "Polarization array"() -> (w679:dbl[])
                              n287 = local write "TimeUp"(FALSE ("TimeUp")) -> ()
                              n288 = call-poly <vilib>:"Mean.vi"("X"=w679) -> ("mean"=w678:dbl)  [unwired: 1 out]
                              n289 = flat-sequence {
                                tunnel: w678 -> [w680]
                                tunnel: [w680] -> w668
                                frame #0 {
                                n290 = local write "Polarization array"(dbl[] [] ("Polarization array")) -> ()
                                }
                              }
                              n291 = Select(t=1, s=w673, f=0) -> (s? t:f=w663:i32)
                              n292 = local read "Actual Field (T)"() -> (w675:dbl)
                              n293 = local read "Averaged P(B)"() -> (w664:dbl[][])
                              n294 = local read "B array"() -> (w672:dbl[])
                              n295 = Index Array(array=w664, index (row)=w663) -> (element=w671:dbl[])  [unwired: 1 in]
                              n296 = local read "Counter"() -> (w667:i8)
                              n297 = Threshold 1D Array(2:w675, 3:w672) -> (0:w662:dbl)  [unwired: 1 in]
                              n298 = Index Array(array=w671, index=w662) -> (element=w670:dbl)
                              "element" <- w670
                              n299 = Increment(x=w667) -> (x+1=w666:i8)
                              n300 = Multiply(x=w667, y=w670) -> (x*y=w669:dbl)
                              n301 = Add(x=w669, y=w668) -> (x+y=w665:dbl)
                              n302 = Divide(x=w665, y=w666) -> (x/y=w661:dbl)
                              n303 = Replace Array Subset(array=w664, new element=w661, index (row)=w663, index (col)=w662) -> (w660:dbl[][])
                              n304 = local write "Averaged P(B)"(w660) -> ()
                              "meanPolarization" <- w668
                            }
                            frame #1 {
                              n305 = local read "Averaged P(B)"() -> (w690:dbl[][])
                              n306 = local read "B array"() -> (w687:dbl[])
                              n307 = Index Array(array=w690, index (row)=1) -> (element=w685:dbl[])  [unwired: 1 in]
                              n308 = Index Array(array=w690, index (row)=0) -> (element=w686:dbl[])  [unwired: 1 in]
                              n309 = Bundle("B array"=w687, "Averaged P(B)"=w686) -> (w684:cluster{"B array":dbl[], "Averaged P(B)":dbl[]})  [unwired: 1 in]
                              n310 = Bundle("B array"=w687, "Averaged P(B)"=w685) -> (w683:cluster{"B array":dbl[], "Averaged P(B)":dbl[]})  [unwired: 1 in]
                              n311 = Build Array(w684, w683) -> (w682:T7)
                              n312 = local write "P(B) /Averaged/"(w682) -> ()
                            }
                          }
                        }
                      }
                    }
                  }
                }
              }
            }
            frame "Plot" {
              # "dI"
              n313 = local read "P(uC/mm^2)"() -> (w692:dbl[])
              n314 = local read "Actual Polarization"() -> (w691:dbl)
              n315 = local read "Actual Current (pA)"() -> (w693:dbl)
              n316 = local read "Time Lag"() -> (w705:dbl)
              n317 = Multiply(x=w693, y=w705) -> (x*y=w697:dbl)
              n318 = Divide(x=w697, y="Sample area (mm^2)") -> (x/y=w696:dbl)
              n319 = Add(x=w696, y=w691) -> (x+y=w695:dbl)
              "Actual Polarization" <- w695
              n320 = local read "Temp/Magnetic Field"() -> (w706:bool)
              n321 = Build Array (concatenate)(w692, w695) -> (→"P(uC/mm^2)":dbl[])
              n322 = case shown="False" w706 {
                tunnel: w703 -> [_ w757]
                tunnel: w700 -> [_ w753]
                tunnel: w695 -> [w713 w754]
                frame False {
                  # "Magnetic Field plotting"
                  n323 = local read "Up/Down"() -> (w718:bool)
                  n324 = case shown="True" w718 {
                    frame True {
                      # "Down"
                      n325 = local read "I(B) 3"() -> (w728:cluster{dbl[], dbl[]}[])
                      n326 = local read "I(B) 3"() -> (w732:cluster{dbl[], dbl[]}[])
                      n327 = Index Array(array=w728, index=1) -> (element=w726:cluster{dbl[], dbl[]})
                      n328 = Unbundle(w726) -> (w725:dbl[], w724:dbl[])
                      n329 = Index Array(array=w732, index=i8 0 ("t")) -> (element=w729:cluster{dbl[], dbl[]})
                      n330 = local read "Actual Current (pA)"() -> (w719:dbl)
                      n331 = local read "Actual B Field (T)"() -> (w721:dbl)
                      n332 = Build Array (concatenate)(w725, w721) -> (w723:dbl[])
                      n333 = Build Array (concatenate)(w724, w719) -> (w722:dbl[])
                      n334 = Bundle(w723, w722) -> (w720:cluster{dbl[], dbl[]})  [unwired: 1 in]
                      n335 = Build Array(w729, w720) -> (w730:cluster{dbl[], dbl[]}[])
                      n336 = local write "I(B) 3"(w730) -> ()
                    }
                    frame False {
                      # "Up"
                      n337 = local read "I(B) 3"() -> (w744:cluster{dbl[], dbl[]}[])
                      n338 = local read "I(B) 3"() -> (w746:cluster{dbl[], dbl[]}[])
                      n339 = Index Array(array=w744, index=0) -> (element=w742:cluster{dbl[], dbl[]})
                      n340 = Unbundle(w742) -> (w741:dbl[], w740:dbl[])
                      n341 = Index Array(array=w746, index=i8 1 ("t")) -> (element=w735:cluster{dbl[], dbl[]})
                      n342 = local read "Actual B Field (T)"() -> (w736:dbl)
                      n343 = Build Array (concatenate)(w741, w736) -> (w739:dbl[])
                      n344 = local read "Actual Current (pA)"() -> (w733:dbl)
                      n345 = Build Array (concatenate)(w740, w733) -> (w738:dbl[])
                      n346 = Bundle(w739, w738) -> (w737:cluster{dbl[], dbl[]})  [unwired: 1 in]
                      n347 = Build Array(w737, w735) -> (w734:cluster{dbl[], dbl[]}[])
                      n348 = local write "I(B) 3"(w734) -> ()
                    }
                  }
                  n349 = local read "Actual B Field (T)"() -> (w715:dbl)
                  n350 = local read "P(B)"() -> (w717:cluster{"yi":dbl[], dbl[]})
                  n351 = Unbundle(w717) -> ("yi"=w716:dbl[], w714:dbl[])
                  n352 = Build Array (concatenate)(w716, w715) -> (w712:dbl[])
                  n353 = Build Array (concatenate)(w714, w713) -> (w711:dbl[])
                  n354 = Bundle(w712, w711) -> (→"P(B)":cluster{dbl[], dbl[]})  [unwired: 1 in]
                }
                frame True {
                  # "Temperature plotting"
                  n355 = local read "Actual Current (pA)"() -> (w756:dbl)
                  n356 = local read "Actual Temperature (K)"() -> (w755:dbl)
                  n357 = local read "Up/Down"() -> (w749:bool)
                  n358 = local read "P(T)"() -> (w750:cluster{dbl[], dbl[]}[])
                  n359 = local read "Sweep"() -> (w752:bool)
                  n360 = local read "I(T)"() -> (w751:cluster{dbl[], dbl[]}[])
                  n361 = case shown="False" w749 {
                    tunnel: w756 -> [w778 w803]
                    tunnel: w755 -> [w774 w799]
                    tunnel: w754 -> [w772 w797]
                    tunnel: w751 -> [w767 w792]
                    tunnel: w750 -> [w762 w789]
                    tunnel: [w763 w790] -> w748
                    tunnel: [w758 w787] -> w747
                    frame True {
                      n362 = Index Array(array=w767, index=1) -> (element=w771:cluster{dbl[], dbl[]})
                      n363 = Index Array(array=w762, index=1) -> (element=w770:cluster{dbl[], dbl[]})
                      n364 = Index Array(array=w762, index=0) -> (element=w759:cluster{dbl[], dbl[]})
                      n365 = Index Array(array=w767, index=0) -> (element=w764:cluster{dbl[], dbl[]})
                      n366 = Unbundle(w770) -> (w775:dbl[], w773:dbl[])
                      n367 = Unbundle(w771) -> (w782:dbl[], w781:dbl[])
                      n368 = Build Array (concatenate)(w775, w774) -> (w776:dbl[])
                      n369 = Build Array (concatenate)(w773, w772) -> (w777:dbl[])
                      n370 = Build Array (concatenate)(w782, w774) -> (w780:dbl[])
                      n371 = Build Array (concatenate)(w781, w778) -> (w779:dbl[])
                      n372 = Bundle(w776, w777) -> (w760:cluster{dbl[], dbl[]})  [unwired: 1 in]
                      n373 = Bundle(w780, w779) -> (w765:cluster{dbl[], dbl[]})  [unwired: 1 in]
                      n374 = Build Array(w759, w760) -> (w758:cluster{dbl[], dbl[]}[])
                      n375 = Build Array(w764, w765) -> (w763:cluster{dbl[], dbl[]}[])
                    }
                    frame False {
                      n376 = Index Array(array=w792, index=0) -> (element=w796:cluster{dbl[], dbl[]})
                      n377 = Index Array(array=w789, index=0) -> (element=w795:cluster{dbl[], dbl[]})
                      n378 = Index Array(array=w789, index=1) -> (element=w783:cluster{dbl[], dbl[]})
                      n379 = Index Array(array=w792, index=1) -> (element=w786:cluster{dbl[], dbl[]})
                      n380 = Unbundle(w795) -> (w800:dbl[], w798:dbl[])
                      n381 = Unbundle(w796) -> (w807:dbl[], w806:dbl[])
                      n382 = Build Array (concatenate)(w800, w799) -> (w801:dbl[])
                      n383 = Build Array (concatenate)(w798, w797) -> (w802:dbl[])
                      n384 = Build Array (concatenate)(w807, w799) -> (w805:dbl[])
                      n385 = Build Array (concatenate)(w806, w803) -> (w804:dbl[])
                      n386 = Bundle(w801, w802) -> (w784:cluster{dbl[], dbl[]})  [unwired: 1 in]
                      n387 = Bundle(w805, w804) -> (w785:cluster{dbl[], dbl[]})  [unwired: 1 in]
                      n388 = Build Array(w784, w783) -> (w787:cluster{dbl[], dbl[]}[])
                      n389 = Build Array(w785, w786) -> (w790:cluster{dbl[], dbl[]}[])
                    }
                  }
                  "I(T)" <- w748
                  "P(T)" <- w747
                  n390 = case shown="False" w752 {
                    tunnel: w757 -> [w812 _]
                    tunnel: w753 -> [w809 _]
                    frame False {
                      n391 = Quotient & Remainder(x=w812, y="Save Period") -> (x-y*floor(x/y)=w808:dbl)  [unwired: 1 out]
                      n392 = Greater?(x=w809, y=w808) -> (0:w810:bool)
                      n393 = case shown="True" w810 {
                        frame False {
                        }
                        frame True {
                          n394 = local write "Reset"(TRUE) -> ()
                        }
                      }
                    }
                    frame True {
                    }
                  }
                }
              }
            }
            frame "Save" {
              n395 = local read "Reset"() -> (w814:bool)
              n396 = case shown="True" w814 {
                tunnel: w819 -> [w836 w838]
                tunnel: [w836 w841] -> w824
                tunnel: w818 -> [w835 w839]
                tunnel: [w835 w841] -> w823
                tunnel: w820 -> [w834 w840]
                tunnel: [w834 w841] -> w822
                tunnel: [w833 w841] -> w821
                tunnel: w817 -> [w833 w837]
                frame False {
                }
                frame True {
                  n397 = stacked-sequence {
                    tunnel: [_ _ w928] -> w841
                    tunnel: w840 -> [_ w923 _]
                    tunnel: w839 -> [w844 w921 _]
                    tunnel: w838 -> [w845 w922 _]
                    tunnel: w837 -> [w843 w919 _]
                    frame #0 {
                      n398 = local read "Temp/Magnetic Field"() -> (w842:bool)
                      n399 = case shown="False" w842 {
                        tunnel: w845 -> [w852 w906]
                        tunnel: w844 -> [w851 w905]
                        tunnel: w843 -> [w849 w896]
                        frame False {
                          n400 = local read "Stepping Mode"() -> (w847:bool)
                          n401 = local read "Up/Down"() -> (w846:bool)
                          n402 = local read "Counter"() -> (w850:i8)
                          n403 = local read "B array"() -> (w848:dbl[])
                          n404 = case shown="False" w847 {
                            tunnel: w852 -> [w880 _]
                            tunnel: w851 -> [w879 _]
                            tunnel: w850 -> [w878 _]
                            tunnel: w849 -> [w870 _]
                            tunnel: w848 -> [w864 _]
                            tunnel: w846 -> [w853 _]
                            frame False {
                              n405 = local read "Averaged I(B)"() -> (w855:dbl[][])
                              n406 = local read "Sample area (mm^2)"() -> (w860:dbl)
                              n407 = call "Average_IBP_curves_baseline.vi"("I in"=w879, "Averaged P(B) In"="Averaged P(B)", "Counter"=w878, "B0"="Threshold B (T)", "Averaged I(B) In"=w855, "t in"=w870, "B in"=w880, "Averaged dt in"="Averaged dt", "Up/Down"=w853, "Sample area(mm^2)"=w860, "B array"=w864) -> ("Averaged dt Out"=w867:dbl[][], "Averaged P(B) Out"=w856:dbl[][], "BaselineSubtracted I(B)"=w854:dbl[][])  [unwired: 1 in, 1 out]
                              "Averaged I(B)" <- w854
                              n408 = Index Array(array=w856, index (row)=0 ("disabled index (col)")) -> (element=w865:dbl[])  [unwired: 1 in]
                              n409 = Index Array(array=w856, index (row)=1 ("disabled index (col)")) -> (element=w866:dbl[])  [unwired: 1 in]
                              n410 = Index Array(array=w854, index (row)=0 ("disabled index (col)")) -> (element=w872:dbl[])  [unwired: 1 in]
                              n411 = Index Array(array=w854, index (row)=1 ("disabled index (col)")) -> (element=w871:dbl[])  [unwired: 1 in]
                              n412 = local write "Averaged dt"(w867) -> ()
                              n413 = Bundle("B array"=w864, "Averaged P(B) Out"=w865) -> (w863:T8)  [unwired: 1 in]
                              n414 = Bundle("B array"=w864, "Averaged P(B) Out"=w866) -> (w862:T8)  [unwired: 1 in]
                              n415 = local write "Averaged P(B)"(w856) -> ()
                              n416 = Bundle("B array"=w864, "BaselineSubtracted I(B)"=w872) -> (w877:T9)  [unwired: 1 in]
                              n417 = Bundle("B array"=w864, "BaselineSubtracted I(B)"=w871) -> (w876:T9)  [unwired: 1 in]
                              n418 = Build Array(w863, w862) -> (→"P(B) /Averaged/":T10)
                              n419 = Build Array(w877, w876) -> (→"I(B) /Averaged/":T11)
                            }
                            frame True {
                            }
                          }
                        }
                        frame True {
                          n420 = local read "T array"() -> (w891:dbl[])
                          n421 = local read "Counter"() -> (w904:i8)
                          n422 = local read "Averaged I(T)"() -> (w883:dbl[][])
                          n423 = local read "Up/Down"() -> (w907:bool)
                          n424 = local read "Averaged dt"() -> (w882:dbl[][])
                          n425 = local read "Sample area (mm^2)"() -> (w887:dbl)
                          n426 = call "Average_ITP_curves.vi"("I in"=w905, "Averaged P(T) In"="Averaged P(T)", "Counter"=w904, "Averaged I(T) In"=w883, "t in"=w896, "T in"=w906, "Averaged dt in"=w882, "Up/Down"=w907, "Sample area(mm^2)"=w887, "T array"=w891) -> ("Averaged I(B) out"=w881:dbl[][], "Averaged dt Out"=w894:dbl[][], "Averaged P(T) Out"=w884:dbl[][])  [unwired: 3 in]
                          "Averaged I(T)" <- w881
                          n427 = Index Array(array=w884, index (row)=0 ("disabled index (col)")) -> (element=w892:dbl[])  [unwired: 1 in]
                          n428 = Index Array(array=w884, index (row)=1 ("disabled index (col)")) -> (element=w893:dbl[])  [unwired: 1 in]
                          n429 = Index Array(array=w881, index (row)=0 ("disabled index (col)")) -> (element=w898:dbl[])  [unwired: 1 in]
                          n430 = Index Array(array=w881, index (row)=1 ("disabled index (col)")) -> (element=w897:dbl[])  [unwired: 1 in]
                          n431 = local write "Averaged dt"(w894) -> ()
                          n432 = Bundle("T array"=w891, "Averaged P(T) Out"=w892) -> (w890:T12)  [unwired: 1 in]
                          n433 = Bundle("T array"=w891, "Averaged P(T) Out"=w893) -> (w889:T12)  [unwired: 1 in]
                          n434 = local write "Averaged P(T)"(w884) -> ()
                          n435 = Bundle("T array"=w891, "Averaged I(B) out"=w898) -> (w903:T13)  [unwired: 1 in]
                          n436 = Bundle("T array"=w891, "Averaged I(B) out"=w897) -> (w902:T13)  [unwired: 1 in]
                          n437 = Build Array(w890, w889) -> (→"P(T) /Averaged/":T14)
                          n438 = Build Array(w903, w902) -> (→"I(T) /Averaged/":T15)
                        }
                      }
                    }
                    frame #1 {
                      # "Save and Reset"
                      n439 = local read "Up/Down"() -> (w909:bool)
                      n440 = local read "Measurement File"() -> (w914:path)
                      n441 = local read "P(uC/mm^2)"() -> (w920:dbl[])
                      n442 = case shown="True" w909 {
                        tunnel: [w925 w926] -> w908
                        frame False {
                          n443 = local read "Measurement File_dn"() -> (w925:path)
                        }
                        frame True {
                          n444 = local read "Measurement File_up"() -> (w926:path)
                        }
                      }
                      n445 = Build Array(w923, w922, w921, w919, w920) -> (w913:dbl[][])
                      n446 = case shown="True" "Reset IB?" {
                        frame False {
                        }
                        frame True {
                          n447 = local read "Up/Down"() -> (w927:bool)
                          n448 = case shown="False" w927 {
                            frame False {
                              n449 = invoke on="I(B) 3" class="XYGraph (strict)" method="Reinit To Default"() -> ()  [unwired: 3 in, 3 out]
                              n450 = invoke on="I(T)" class="XYGraph (strict)" method="Reinit To Default"() -> ()  [unwired: 3 in, 3 out]
                            }
                            frame True {
                            }
                          }
                        }
                      }
                      n451 = call-poly <vilib>:"Write Delimited Spreadsheet.vi"("file path (dialog if empty)"=w914, "format (%.3f)"="%.5g", "2D data"=w913, "append to file? (F)"=TRUE, "transpose? (F)"=TRUE) -> ()  [unwired: 9 in, 2 out]
                      n452 = call-poly <vilib>:"Write Delimited Spreadsheet.vi"("file path (dialog if empty)"=w908, "format (%.3f)"="%.5g", "2D data"=w913, "append to file? (F)"=TRUE ("transpose? (F)"), "transpose? (F)"=FALSE ("append to file? (F)")) -> ()  [unwired: 9 in, 2 out]
                      n453 = local write "Reset"(FALSE ("Save")) -> ()
                    }
                    frame #2 {
                      w928 = dbl[] []
                      n454 = local write "P(uC/mm^2)"(w928) -> ()
                    }
                  }
                }
              }
              n455 = local read "New"() -> (w816:bool)
              n456 = case shown="False" w816 {
                tunnel: [Mode."Return" ("Enum") Mode."New" ("Enum")] -> w828
                tunnel: [TRUE FALSE] -> w815
                frame False {
                }
                frame True {
                }
              }
            }
            frame "New" {
              n457 = stacked-sequence {
                seq-local: [_ _ _ _ w1076 _ _] -> [_ _ _ _ _ w1093 _]
                seq-local: [_ _ w1013 _ _ _ _] -> [_ _ _ w1049 _ _ _]
                seq-local: [_ _ _ w1048 _ _ _] -> [_ _ _ _ w1074 _ _]
                seq-local: [_ w968 _ _ _ _ _] -> [_ _ w1007 _ _ _ _]
                tunnel: T6 {"Com Port"=1, "ISOBUS Address"=0, "GPIB Address"=25, "Communication"=enum."GPIB"} ("Address") -> [_ _ w1012 w1054 _ _ _]
                tunnel: w931 -> [_ w969 _ _ _ w1094 _]
                tunnel: [_ _ _ _ _ w1096 _] -> w930
                tunnel: w929 -> [_ w972 _ _ _ _ _]
                frame #0 {
                  w958 = 1 ("index (row)")
                  w957 = 0 ("index (row)")
                  # "Save averages"
                  n458 = local read "Temp/Magnetic Field"() -> (w941:bool)
                  n459 = case shown="True" w941 {
                    tunnel: [w965 w966] -> w956
                    tunnel: [w964 w967] -> w946
                    frame False {
                      n460 = local read "Averaged P(B)"() -> (w965:dbl[][])
                      n461 = local read "I(B) /Averaged/"() -> (w964:cluster{"B array":dbl[], dbl[]}[])
                    }
                    frame True {
                      n462 = local read "Averaged P(T)"() -> (w966:dbl[][])
                      n463 = local read "I(T) /Averaged/"() -> (w967:cluster{"B array":dbl[], dbl[]}[])
                    }
                  }
                  n464 = local read "Measurement File_average"() -> (w945:path)
                  n465 = local read "Averaged dt"() -> (w954:dbl[][])
                  n466 = Index Array(array=w954, index (row)=w957) -> (element=w955:dbl[])  [unwired: 1 in]
                  n467 = Index Array(array=w954, index (row)=w958) -> (element=w962:dbl[])  [unwired: 1 in]
                  n468 = Index Array(array=w946, index=1) -> (element=w950:cluster{"B array":dbl[], dbl[]})
                  n469 = Index Array(array=w946, index=0) -> (element=w949:cluster{"B array":dbl[], dbl[]})
                  n470 = Unbundle(w950) -> ("B array"=w960:dbl[], w961:dbl[])
                  n471 = Unbundle(w949) -> ("B array"=w951:dbl[], w952:dbl[])
                  n472 = Index Array(array=w956, index (row)=w957) -> (element=w959:dbl[])  [unwired: 1 in]
                  n473 = Index Array(array=w956, index (row)=w958) -> (element=w963:dbl[])  [unwired: 1 in]
                  n474 = Build Array(w951, w952, w955, w959, w960, w961, w962, w963) -> (w953:dbl[][])
                  n475 = call-poly <vilib>:"Write Delimited Spreadsheet.vi"("file path (dialog if empty)"=w945, "format (%.3f)"="%.5g", "2D data"=w953, "append to file? (F)"=TRUE ("transpose? (F)"), "transpose? (F)"=TRUE ("append to file? (F)")) -> ()  [unwired: 9 in, 2 out]
                }
                frame #1 {
                  w980 = dbl[] []
                  # "Reset Flags"
                  n476 = Get Date/Time In Seconds() -> (seconds since 1Jan1904=w981:timestamp)
                  n477 = local write "Measuring"(FALSE ("Measuring")) -> ()
                  n478 = local write "Up/Down"(TRUE ("Up/Down")) -> ()
                  n479 = local write "First?"(TRUE ("First?")) -> ()
                  n480 = local write "Offset?"(FALSE ("Offset?")) -> ()
                  n481 = local write "New"(FALSE ("New")) -> ()
                  n482 = local write "P(uC/mm^2)"(w980) -> ()
                  n483 = local write "Start time"(w981) -> ()
                  n484 = local write "Offset array"(w980) -> ()
                  n485 = local write "Actual Polarization"(0.0 ("Actual Polarization")) -> ()
                  n486 = local write "Up/Down"(TRUE ("Up/Down")) -> ()
                  n487 = local read "Temp/Magnetic Field"() -> (w970:bool)
                  n488 = local write "Reset"(FALSE ("Reset")) -> ()
                  n489 = case shown="False" w970 {
                    tunnel: w969 -> [w986 w999]
                    tunnel: [w984 w999] -> w968
                    frame True {
                      w992 = dbl[] []
                      n490 = local read "B array"() -> (w994:dbl[])
                      n491 = invoke on="I(T)" class="XYGraph (strict)" method="Reinit To Default"() -> ()  [unwired: 3 in, 3 out]
                      n492 = Build Array(w992, w992) -> (w998:dbl[][])
                      n493 = Multiply(x=w994, y=0.0) -> (x*y=w995:dbl[])
                      n494 = Bundle("B array"=w994, w995) -> (w996:cluster{"B array":dbl[], dbl[]})  [unwired: 1 in]
                      n495 = local write "Averaged I(T)"(w998) -> ()
                      n496 = invoke on="P(T)" class="XYGraph (strict)" method="Reinit To Default"() -> ()  [unwired: 3 in, 3 out]
                      n497 = Build Array(w996, w996) -> (w997:cluster{"B array":dbl[], dbl[]}[])
                      n498 = local write "I(T) /Averaged/"(w997) -> ()
                      n499 = local read "Set temperature (K)"() -> (w991:dbl)
                      n500 = Number To Fractional String(number=w991, precision (6)=i16 3) -> (F-format string=w988:string)  [unwired: 2 in]
                      n501 = local read "Lake Shore"() -> (w985:refnum<visa-resource-name>)
                      n502 = Concatenate Strings("SETP 1," ("write buffer"), w988) -> (w990:string)
                      n503 = VISA Write(VISA resource name=w985, write buffer=w990, error in (no error)=w986) -> (error out=w984:errorcluster)  [unwired: 2 out]
                    }
                    frame False {
                      w1000 = dbl[] []
                      n504 = local read "B array"() -> (w1002:dbl[])
                      n505 = invoke on="I(B) 3" class="XYGraph (strict)" method="Reinit To Default"() -> ()  [unwired: 3 in, 3 out]
                      n506 = Build Array(w1000, w1000) -> (w1006:dbl[][])
                      n507 = Multiply(x=w1002, y=0.0) -> (x*y=w1003:dbl[])
                      n508 = Bundle("B array"=w1002, w1003) -> (w1004:cluster{"B array":dbl[], dbl[]})  [unwired: 1 in]
                      n509 = local write "Averaged I(B)"(w1006) -> ()
                      n510 = invoke on="P(B)" class="XYGraph (strict)" method="Reinit To Default"() -> ()  [unwired: 3 in, 3 out]
                      n511 = Build Array(w1004, w1004) -> (w1005:cluster{"B array":dbl[], dbl[]}[])
                      n512 = local write "I(B) /Averaged/"(w1005) -> ()
                    }
                  }
                  n513 = local write "Counter"(i8 0 ("Counter")) -> ()
                  n514 = Flush Queue(queue=w972) -> (remaining elements=→"remaining elements 2":T1)  [unwired: 1 in, 2 out]
                }
                frame #2 {
                  # "Step"
                  n515 = local read "Sweep Rate Array"() -> (w1010:dbl[])
                  n516 = local read "T Sweep Rate Array"() -> (w1011:dbl[])
                  n517 = local read "Temp/Magnetic Field"() -> (w1008:bool)
                  n518 = local read "j"() -> (w1017:i32)
                  n519 = Increment(x=w1017) -> (x+1=w1014:i32)
                  n520 = Select(t=w1011, s=w1008, f=w1010) -> (s? t:f=w1009:dbl[])
                  n521 = Array Size(array=w1009) -> (size(s)=w1016:i32)
                  n522 = Less?(x=w1014, y=w1016) -> (x < y?=w1015:bool)
                  "Step Rate" <- w1015
                  n523 = case shown="False" w1015 {
                    tunnel: w1014 -> [_ w1047]
                    tunnel: w1007 -> [w1024 w1046]
                    tunnel: [w1023 w1046] -> w1013
                    tunnel: w1012 -> [w1022 _]
                    tunnel: w1008 -> [w1020 _]
                    frame False {
                      # "Step Temp?"
                      n524 = local read "Magnetic Field array (T)"() -> (w1019:dbl[])
                      n525 = local read "Temperature Array"() -> (w1021:dbl[])
                      n526 = local read "i"() -> (w1028:i32)
                      n527 = Select(t=w1019, s=w1020, f=w1021) -> (s? t:f=w1018:dbl[])
                      n528 = Increment(x=w1028) -> (x+1=w1026:i32)
                      n529 = local write "j"(0 ("f")) -> ()
                      n530 = Array Size(array=w1018) -> (size(s)=w1027:i32)
                      n531 = Less?(x=w1026, y=w1027) -> (x < y?=w1025:bool)
                      "Step Temp" <- w1025
                      n532 = case shown="True" w1025 {
                        tunnel: w1026 -> [_ w1045]
                        tunnel: w1024 -> [w1033 w1044]
                        tunnel: [w1032 w1044] -> w1023
                        tunnel: w1022 -> [w1031 _]
                        frame False {
                          # "Heater OFF"
                          # "Finished"
                          n533 = local write "i"(0 ("i")) -> ()
                          n534 = stacked-sequence {
                            tunnel: w1033 -> [w1037 _ _]
                            tunnel: [w1036 _ _] -> w1032
                            tunnel: w1031 -> [_ w1041 w1042]
                            frame #0 {
                              n535 = local read "Lake Shore"() -> (w1038:refnum<visa-resource-name>)
                              n536 = VISA Write(VISA resource name=w1038, write buffer="RANGE,1,0", error in (no error)=w1037) -> (error out=w1036:errorcluster)  [unwired: 2 out]
                            }
                            frame #1 {
                              n537 = call "ips_switchHeaterOff.vi"("Instrument address"=w1041, "Rate"=2.0) -> ()  [unwired: 1 out]
                            }
                            frame #2 {
                              n538 = call "GPIB - BusCommand.vi"("Command"="H0", "Address"=w1042) -> ()  [unwired: 2 out]
                            }
                          }
                          n539 = local write "Record ALL"(FALSE ("Record ALL")) -> ()
                          "Finished" <- TRUE
                        }
                        frame True {
                          n540 = local write "i"(w1045) -> ()
                        }
                      }
                    }
                    frame True {
                      n541 = local write "j"(w1047) -> ()
                    }
                  }
                }
                frame #3 {
                  # "Set rates"
                  n542 = local read "Temp/Magnetic Field"() -> (w1051:bool)
                  n543 = local read "Max count array"() -> (w1050:i32[])
                  n544 = local read "j"() -> (w1053:i32)
                  n545 = case shown="True" w1051 {
                    tunnel: w1054 -> [w1059 _]
                    tunnel: w1049 -> [w1055 w1066]
                    tunnel: [w1055 w1065] -> w1048
                    frame False {
                      n546 = local read "Sweep Rate Array"() -> (w1058:dbl[])
                      n547 = local read "j"() -> (w1057:i32)
                      n548 = Index Array(array=w1058, index=w1057) -> (element=w1056:dbl)
                      n549 = Number To Fractional String(number=w1056, precision (6)=i16 3) -> (F-format string=w1062:string)  [unwired: 2 in]
                      n550 = Concatenate Strings("T" ("format string"), w1062) -> (w1063:string)
                      n551 = call "GPIB - BusCommand.vi"("Command"=w1063, "Address"=w1059) -> ()  [unwired: 2 out]
                      n552 = local write "Sweep Rate (T/min)"(w1056) -> ()
                    }
                    frame True {
                      n553 = local read "T Sweep Rate Array"() -> (w1072:dbl[])
                      n554 = local read "j"() -> (w1073:i32)
                      n555 = Index Array(array=w1072, index=w1073) -> (element=w1068:dbl)
                      n556 = Number To Fractional String(number=w1068, precision (6)=i16 1) -> (F-format string=w1070:string)  [unwired: 2 in]
                      n557 = local read "Lake Shore"() -> (w1064:refnum<visa-resource-name>)
                      n558 = local write "Temp Ramping Rate (K/min)"(w1068) -> ()
                      n559 = Concatenate Strings("RAMP 1,1," ("string"), w1070) -> (w1071:string)
                      n560 = VISA Write(VISA resource name=w1064, write buffer=w1071, error in (no error)=w1066) -> (error out=w1065:errorcluster)  [unwired: 2 out]
                    }
                  }
                  n561 = Index Array(array=w1050, index=w1053) -> (element=w1052:i32)
                  n562 = local write "Max Countl"(w1052) -> ()
                }
                frame #4 {
                  # "Set temperature/Field"
                  n563 = local read "Temp/Magnetic Field"() -> (w1075:bool)
                  n564 = case shown="True" w1075 {
                    tunnel: [w1077 w1084] -> w1076
                    tunnel: w1074 -> [w1078 w1083]
                    frame True {
                      n565 = local read "Magnetic Field array (T)"() -> (w1081:dbl[])
                      n566 = local read "i"() -> (w1082:i32)
                      n567 = Index Array(array=w1081, index=w1082) -> (element=w1079:dbl)
                      n568 = call "Set_B.vi"("error in (no error)"=w1078, "address string"="25", "Set Field (T)"=w1079) -> ("error out"=w1077:errorcluster)  [unwired: 8 in]
                    }
                    frame False {
                      n569 = local read "Temperature Array"() -> (w1087:dbl[])
                      n570 = local read "i"() -> (w1086:i32)
                      n571 = Index Array(array=w1087, index=w1086) -> (element=w1085:dbl)
                      n572 = local read "Lake Shore"() -> (w1089:refnum<visa-resource-name>)
                      n573 = Number To Fractional String(number=w1085, precision (6)=i16 3) -> (F-format string=w1090:string)  [unwired: 2 in]
                      n574 = Concatenate Strings("SETP 1," ("write buffer"), w1090) -> (w1092:string)
                      n575 = VISA Write(VISA resource name=w1089, write buffer=w1092, error in (no error)=w1083) -> (error out=w1084:errorcluster)  [unwired: 2 out]
                    }
                  }
                }
                frame #5 {
                  n576 = local read "Finished"() -> (w1095:bool)
                  n577 = case shown="False" w1095 {
                    tunnel: [w1124 w1157] -> w1096
                    tunnel: w1094 -> [_ _]
                    tunnel: w1093 -> [w1121 w1157]
                    frame False {
                      w1119 = "_" ("string")
                      # "Wait, create Files"
                      n578 = local read "Magnetic Field array (T)"() -> (w1106:dbl[])
                      n579 = local read "Temp/Magnetic Field"() -> (w1098:bool)
                      n580 = local read "Temperature Array"() -> (w1111:dbl[])
                      n581 = local read "T Sweep Rate Array"() -> (w1108:dbl[])
                      n582 = local read "Sweep Rate Array"() -> (w1109:dbl[])
                      n583 = local read "i"() -> (w1147:i32)
                      n584 = local read "j"() -> (w1145:i32)
                      n585 = Select(t=w1108, s=w1098, f=w1109) -> (s? t:f=w1107:dbl[])
                      n586 = Index Array(array=w1107, index=w1145) -> (element=w1116:dbl)
                      n587 = Round Toward -Infinity(1:w1116) -> (0:w1117:dbl)
                      n588 = Multiply(x=w1106, y=i16 1000 ("precision (6)")) -> (x*y=w1104:dbl[])
                      n589 = Select(t=w1104, s=w1098, f=w1111) -> (s? t:f=w1110:dbl[])
                      n590 = Index Array(array=w1110, index=w1147) -> (element=w1146:dbl)
                      n591 = Number To Fractional String(use system decimal point (T)=TRUE, number=w1146, precision (6)=i16 1) -> (F-format string=w1148:string)  [unwired: 1 in]
                      n592 = Subtract(x=w1116, y=w1117) -> (x-y=w1118:dbl)
                      n593 = Equal To 0?(x=w1118) -> (x = 0?=w1115:bool)
                      n594 = Select(t="mT" ("string"), s=w1098, f="K" ("string")) -> (s? t:f=w1101:string)
                      n595 = Select(t=i16 0 ("precision (6)"), s=w1115, f=i16 2 ("precision (6)")) -> (s? t:f=w1112:i16)
                      n596 = Number To Fractional String(use system decimal point (T)=TRUE, number=w1116, precision (6)=w1112) -> (F-format string=w1120:string)  [unwired: 1 in]
                      n597 = Select(t="Kpm" ("string"), s=w1098, f="Tpm" ("string")) -> (s? t:f=w1097:string)
                      n598 = Concatenate Strings("Directory", "\\" ("string"), "FileName", w1119, w1148, w1101, w1119, w1120, w1097) -> (w1141:string)
                      n599 = Search and Replace String(replace all?=TRUE ("replace all? (F)"), input string=w1141, search string=".", replace string="p" ("substring (\"\")"), error in=w1121) -> (result string=w1136:string, error out=w1131:errorcluster)  [unwired: 3 in, 2 out]
                      n600 = local write "Step Rate"(FALSE ("Step Rate")) -> ()
                      n601 = Concatenate Strings(w1136, ".txt" ("string")) -> (w1135:string)
                      n602 = local read "Step Temp"() -> (w1125:bool)
                      n603 = String To Path(string=w1135) -> (path=w1134:path)
                      n604 = Open/Create/Replace File(file path (use dialog)=w1134, error in=w1131, operation (0:open)=T5."open or create") -> (refnum out=w1123:refnum<file>, error out=w1124:errorcluster)  [unwired: 3 in, 1 out]
                      n605 = local write "refnum out"(w1123) -> ()
                      n606 = Refnum to Path(1:w1123) -> (0:w1126:path)
                      n607 = call "Create_sweep_files.vi"("Measurement File"=w1126) -> ("Path 3"=w1129:path, "Path 2"=w1128:path, "Path"=w1127:path)  [unwired: 8 in]
                      n608 = local write "Measurement File"(w1126) -> ()
                      n609 = case shown="True" w1125 {
                        frame False {
                        }
                        frame True {
                          n610 = Get Date/Time In Seconds() -> (seconds since 1Jan1904=w1150:timestamp)
                          n611 = local write "Step Temp"(FALSE ("Step Temp")) -> ()
                          n612 = while {
                            tunnel: w1150 -> [w1155]
                            stop <- w1152 stop-if-true
                            n613 = Get Date/Time In Seconds() -> (seconds since 1Jan1904=w1156:timestamp)
                            n614 = Subtract(x=w1156, y=w1155) -> (x-y=w1154:dbl)
                            "Wait (s)" <- w1154
                            n615 = Greater Or Equal?(x=w1154, y="secs to wait") -> (x >= y?=w1152:bool)
                          }
                        }
                      }
                      n616 = local write "Measurement File_dn"(w1129) -> ()
                      n617 = local write "Measurement File_average"(w1127) -> ()
                      n618 = local write "Measurement File_up"(w1128) -> ()
                    }
                    frame True {
                    }
                  }
                }
                frame #6 {
                  n619 = local read "Finished"() -> (w1158:bool)
                  n620 = case shown="True" w1158 {
                    frame False {
                      n621 = local write "Measuring"(TRUE ("Measuring")) -> ()
                    }
                    frame True {
                      n622 = local write "Measure /Pause"(FALSE ("Measure /Pause")) -> ()
                    }
                  }
                }
              }
            }
            frame "Return" {
            }
          }
        }
      }
      frame Error {
        # "Return true for any case which should stop the loop."
      }
    }
  }
  n623 = VISA Read(VISA resource name=w27, byte count=u32 100, error in (no error)=w29) -> (VISA resource name out=w26:refnum<visa-resource-name>, read buffer=w25:string, error out=w28:errorcluster)  [unwired: 1 out]
  n624 = VISA Open(error in (no error)=w28, VISA resource name="Magnetic Field") -> (VISA resource name=w120:refnum<visa-resource-name>, error out=w102:errorcluster)  [unwired: 3 in]
  n625 = VISA Open(error in (no error)=w102, VISA resource name="Lake Shore") -> (VISA resource name=w97:refnum<visa-resource-name>, error out=w68:errorcluster)  [unwired: 3 in]
  n626 = VISA Write(VISA resource name="Lake Shore", write buffer="KRDG?a", error in (no error)=w68) -> (VISA resource name out=w65:refnum<visa-resource-name>, error out=w64:errorcluster)  [unwired: 1 out]
  n627 = VISA Read(VISA resource name=w65, byte count=w71, error in (no error)=w64) -> (VISA resource name out=w62:refnum<visa-resource-name>, read buffer=w76:string, error out=w63:errorcluster)  [unwired: 1 out]
  n628 = VISA Write(VISA resource name=w62, write buffer="SETP?a", error in (no error)=w63) -> (VISA resource name out=w61:refnum<visa-resource-name>, error out=w60:errorcluster)  [unwired: 1 out]
  n629 = VISA Read(VISA resource name=w61, byte count=w71, error in (no error)=w60) -> (VISA resource name out=w58:refnum<visa-resource-name>, read buffer=w75:string, error out=w59:errorcluster)  [unwired: 1 out]
  n630 = VISA Write(VISA resource name=w58, write buffer="RANGE?a", error in (no error)=w59) -> (VISA resource name out=w56:refnum<visa-resource-name>, error out=w57:errorcluster)  [unwired: 1 out]
  n631 = Fract/Exp String To Number(string=w76) -> (number=w74:dbl)  [unwired: 3 in, 1 out]
  n632 = VISA Read(VISA resource name=w56, byte count=w71, error in (no error)=w57) -> (read buffer=w70:string, error out=w67:errorcluster)  [unwired: 2 out]
  n633 = Fract/Exp String To Number(string=w75) -> (number=w73:dbl)  [unwired: 3 in, 1 out]
  n634 = Fract/Exp String To Number(string=w70) -> (number=w66:dbl)  [unwired: 3 in, 1 out]
  n635 = local write "Actual Temperature (K)"(w74) -> ()
  n636 = local write "Setpoint Temperature (K)"(w73) -> ()
  n637 = local write "Heater Range"(w66) -> ()
  n638 = case shown="True" w81 {
    frame False {
    }
    frame True {
      n639 = invoke on="I(B) 3" class="XYGraph (strict)" method="Reinit To Default"() -> ()  [unwired: 3 in, 3 out]
      n640 = invoke on="I(B) /Averaged/" class="XYGraph (strict)" method="Reinit To Default"() -> ()  [unwired: 3 in, 3 out]
      n641 = invoke on="P(T)" class="XYGraph (strict)" method="Reinit To Default"() -> ()  [unwired: 3 in, 3 out]
      n642 = invoke on="P(B)" class="XYGraph (strict)" method="Reinit To Default"() -> ()  [unwired: 3 in, 3 out]
      n643 = invoke on="I(T)" class="XYGraph (strict)" method="Reinit To Default"() -> ()  [unwired: 3 in, 3 out]
      n644 = invoke on="P(B) /Averaged/" class="XYGraph (strict)" method="Reinit To Default"() -> ()  [unwired: 3 in, 3 out]
    }
  }
  n645 = Decimal String To Number(string=w25) -> (number=w24:i32)  [unwired: 2 in, 1 out]
  n646 = local write "Keithley (IV conv) averaging"(w24) -> ()
  n647 = local read "Stepping Mode"() -> (w4:bool)
  n648 = while {
    shift-right: [w1189] -> w118
    shift-left: w99 -> [w1190]
    shift-right: [w1191] -> w123
    shift-left: w124 -> [w1192]
    tunnel: w26 -> [w1188]
    tunnel: w120 -> [w1187]
    tunnel: w67 -> [_]
    tunnel: [w1181] -> _
    tunnel: w107 -> [w1180]
    tunnel: w97 -> [w1179]
    tunnel: w34 -> [w1178]
    stop <- "stop" stop-if-true
    n649 = event shown="[0] Timeout" {
      selector: _ -> [_ _ _ _ _ _ _ _ _ _ _ _ _ _ _ _]
      dyn-events: _ -> [_ _ _ _ _ _ _ _ _ _ _ _ _ _ _ _]
      timeout: 10 -> [_ _ _ _ _ _ _ _ _ _ _ _ _ _ _ _]
      tunnel: w1192 -> [w1202 w1248 w1266 w1276 w1290 w1361 w1365 w1369 w1425 w1441 w1458 w1501 w1518 w1542 w1544 w1555]
      tunnel: [w1201 w1248 w1266 w1276 w1290 w1361 w1365 w1369 w1425 w1441 w1458 w1501 w1518 w1542 w1544 w1555] -> w1191
      tunnel: w1190 -> [w1200 w1257 w1265 w1275 w1288 w1360 w1367 w1371 w1426 w1440 w1457 w1502 w1520 w1536 w1548 w1557]
      tunnel: [w1199 w1249 w1265 w1275 w1287 w1362 w1367 w1370 _ w1440 w1457 w1502 w1519 w1535 w1547 w1556] -> w1189
      tunnel: w1188 -> [w1198 w1258 _ _ _ _ _ _ _ _ _ _ _ _ _ _]
      tunnel: w1187 -> [w1197 _ _ _ _ _ _ _ _ _ _ _ _ _ _ _]
      tunnel: [w1195 w1247 w1264 w1274 w1289 w1363 w1366 w1368 w1424 w1439 w1456 w1500 w1517 w1543 w1545 _] -> w1181
      tunnel: w1180 -> [w1195 w1247 w1264 w1277 w1289 w1363 w1366 w1368 w1424 w1439 w1456 w1500 w1517 w1543 w1545 _]
      tunnel: w1179 -> [_ _ _ _ _ _ _ _ _ _ _ _ w1521 w1534 w1549 w1554]
      tunnel: [_ _ _ _ _ _ _ _ w1426 _ _ _ _ _ _ _] -> _
      tunnel: w1178 -> [w1194 _ _ _ _ _ _ _ _ _ _ _ _ _ _ _]
      event Timeout {
        n650 = event-data() -> ()  [unwired: 1 in, 3 out]
        n651 = case shown="True" "Measuring" {
          tunnel: w1202 -> [w1204 w1227]
          tunnel: [w1204 w1226] -> w1201
          tunnel: w1200 -> [w1203 w1205]
          tunnel: [w1203 w1225] -> w1199
          tunnel: w1198 -> [_ w1218]
          tunnel: w1197 -> [_ w1217]
          tunnel: w1194 -> [_ w1208]
          frame False {
          }
          frame True {
            w1216 = ":FETCh? " ("data")
            w1219 = u32 1000 ("byte count")
            # "Generate the data here."
            n652 = case shown="No Error" w1205 {
              selector: w1205 -> [w1239 w1240]
              tunnel: [w1239 w1240] -> w1213
              tunnel: [w1238 _] -> w1212
              frame No Error {
                n653 = Get Date/Time In Seconds() -> (seconds since 1Jan1904=w1238:timestamp)
              }
              frame Error {
              }
            }
            n654 = VISA Write(VISA resource name=w1218, write buffer=w1216, error in (no error)=w1213) -> (VISA resource name out=w1224:refnum<visa-resource-name>, error out=w1222:errorcluster)  [unwired: 1 out]
            n655 = VISA Write(VISA resource name=w1217, write buffer=w1216, error in (no error)=w1222) -> (VISA resource name out=w1223:refnum<visa-resource-name>, error out=w1221:errorcluster)  [unwired: 1 out]
            n656 = VISA Read(VISA resource name=w1224, byte count=w1219, error in (no error)=w1221) -> (read buffer=w1214:string, error out=w1220:errorcluster)  [unwired: 2 out]
            n657 = VISA Read(VISA resource name=w1223, byte count=w1219, error in (no error)=w1220) -> (read buffer=w1215:string, error out=w1210:errorcluster)  [unwired: 2 out]
            n658 = case shown="False" "DaQ" {
              tunnel: w1210 -> [w1229 w1235]
              tunnel: [w1229 w1234] -> w1209
              tunnel: w1208 -> [_ w1233]
              tunnel: [0.0 ("Output") w1231] -> w1206
              frame False {
              }
              frame True {
                n659 = local read "Number of Samples"() -> (w1237:i32)
                n660 = call-poly <vilib>:"DAQmx Read.vi"("task/channels in"=w1233, "number of samples per channel"=w1237, "error in"=w1235) -> ("data"=w1236:dbl[], "error out"=w1234:errorcluster)  [unwired: 10 in, 1 out]
                n661 = call-poly <vilib>:"Mean.vi"("X"=w1236) -> ("mean"=w1232:dbl)  [unwired: 1 out]
                "Actual mean" <- w1232
                n662 = call "N Point Running Average.vi"("n"="Moving average", "Input"=w1232) -> ("Output"=w1231:dbl)
              }
            }
            n663 = Bundle("seconds since 1Jan1904"=w1212, "read buffer"=w1214, "read buffer"=w1215, "Output"=w1206) -> (w1211:T4)  [unwired: 1 in]
            n664 = Enqueue Element(queue=w1227, element=w1211, error in (no error)=w1209) -> (queue out=w1226:refnum<queue>, error out=w1225:errorcluster)  [unwired: 1 in, 1 out]
          }
        }
      }
      event "Keithley (IV conv) averaging": Value Change {
        n665 = event-data() -> ()  [unwired: 1 in, 6 out]
        n666 = Number To Decimal String(number="Keithley (IV conv) averaging") -> (decimal integer string=w1255:string)  [unwired: 1 in]
        n667 = Concatenate Strings("VOLTage:DC:AVERage:COUNt " ("write buffer"), w1255) -> (w1254:string)
        n668 = VISA Write(VISA resource name=w1258, write buffer=w1254, error in (no error)=w1257) -> (VISA resource name out=w1253:refnum<visa-resource-name>, error out=w1251:errorcluster)  [unwired: 1 out]
        n669 = VISA Write(VISA resource name=w1253, write buffer="VOLTage:DC:AVERage:COUNt?", error in (no error)=w1251) -> (VISA resource name out=w1246:refnum<visa-resource-name>, error out=w1250:errorcluster)  [unwired: 1 out]
        n670 = VISA Read(VISA resource name=w1246, byte count=u32 100, error in (no error)=w1250) -> (read buffer=w1244:string, error out=w1249:errorcluster)  [unwired: 2 out]
        n671 = Decimal String To Number(string=w1244) -> (number=w1243:i32)  [unwired: 2 in, 1 out]
        n672 = Equal?(x="Keithley (IV conv) averaging", y=w1243) -> (x = y?=→"Confirm":bool)
      }
      event "Max Field (T)": Value Change {
        n673 = event-data() -> ()  [unwired: 1 in, 6 out]
        n674 = Divide(x="Max Field (T)", y="dB (T)") -> (x/y=w1261:dbl)
        n675 = for {
          N: w1261 -> [_]
          tunnel: "dB (T)" -> [w1271]
          tunnel: [w1268] -> w1260 mode=indexing
          tunnel: "Min Field (T)" -> [w1269]
          tunnel: [0.0] -> _ mode=indexing
          i -> [w1272]
          n676 = Multiply(x=w1272, y=w1271) -> (x*y=w1270:dbl)
          n677 = Add(x=w1270, y=w1269) -> (x+y=w1268:dbl)
        }
        "B array" <- w1260
      }
      event "Sweep Rate (T/min)": Value Change {
        n678 = event-data() -> ("NewVal"=w1278:dbl)  [unwired: 1 in, 5 out]
        n679 = local read "Magnet"() -> (w1273:bool)
        n680 = case shown="False" w1273 {
          tunnel: w1278 -> [_ w1285]
          tunnel: w1277 -> [w1279 w1281]
          tunnel: [w1279 w1280] -> w1274
          frame False {
          }
          frame True {
            n681 = Number To Fractional String(number=w1285, precision (6)=i16 3) -> (F-format string=w1283:string)  [unwired: 2 in]
            n682 = Concatenate Strings("T" ("format string"), w1283) -> (w1282:string)
            n683 = call "GPIB - BusCommand.vi"("Command"=w1282, "Address"=w1281) -> ("Address(thru)"=w1280:T6)  [unwired: 1 out]
          }
        }
      }
      event "Field To Zero": Value Change {
        n684 = event-data() -> ()  [unwired: 1 in, 6 out]
        n685 = Two Button Dialog(message="Do you want to switch off the field?", 1:"No" ("F button name (\"Cancel\")"), 2:"Yes" ("T button name (\"OK\")")) -> (T button?=w1294:bool)
        n686 = case shown="True" w1294 {
          tunnel: w1289 -> [_ w1299]
          tunnel: w1288 -> [w1295 w1297]
          tunnel: [w1295 w1296] -> w1287
          frame False {
          }
          frame True {
            n687 = local read "Magnet"() -> (w1298:bool)
            n688 = case shown="False" w1298 {
              tunnel: w1299 -> [_ w1351]
              tunnel: w1297 -> [w1302 w1348]
              tunnel: [w1301 w1348] -> w1296
              frame False {
                n689 = local read "Lock_in_Amplifier"() -> (w1300:refnum<visa-resource-name>)
                n690 = stacked-sequence {
                  seq-local: [w1305 _] -> [_ w1317]
                  seq-local: [w1303 _] -> [_ w1314]
                  tunnel: w1302 -> [w1307 _]
                  tunnel: [_ w1320] -> w1301
                  tunnel: w1300 -> [w1304 w1315]
                  frame #0 {
                    n691 = VISA Write(VISA resource name=w1304, write buffer="AUXV?1", error in (no error)=w1307) -> (VISA resource name out=w1311:refnum<visa-resource-name>, error out=w1306:errorcluster)  [unwired: 1 out]
                    n692 = VISA Read(VISA resource name=w1311, byte count=u32 1000, error in (no error)=w1306) -> (read buffer=w1308:string, error out=w1305:errorcluster)  [unwired: 2 out]
                    n693 = Fract/Exp String To Number(string=w1308) -> (number=w1303:dbl)  [unwired: 3 in, 1 out]
                  }
                  frame #1 {
                    w1323 = 0.001 ("Voltage Step (V)")
                    n694 = local read "Sweep Rate (T/min)"() -> (w1322:dbl)
                    n695 = local read "V/I (Ohm)"() -> (w1319:dbl)
                    n696 = local read "B/V (T/V)"() -> (w1313:dbl)
                    n697 = xnode "Sweep Delay"("SweepRate"=w1322, "Resolution"=w1323, "BpV"=w1313) -> ("Result"=w1321:dbl)  [unwired: 1 in, 1 out]
                    n698 = call "Universal_Ramping.vi"("milliseconds to wait"=w1321, "Initial Voltage (V)"=w1314, "error in (no error)"=w1317, "Voltage Step (V)"=w1323, "Final Voltage (V)"=0.0, "VISA resource name"=w1315) -> ("error out"=w1320:errorcluster, "Actual Voltage (V)"=w1312:dbl)  [unwired: 3 in, 1 out]
                    n699 = local write "Actual Voltage (V)"(w1312) -> ()
                    n700 = xnode "AUXtoB"("BpV"=w1313, "Rm"=w1319, "Aux"=w1312) -> ("Result"=w1318:dbl)  [unwired: 1 in, 1 out]
                    n701 = local write "Actual B Field (T)"(w1318) -> ()
                  }
                }
              }
              frame True {
                n702 = local read "Sweep Rate (T/min)"() -> (w1350:dbl)
                n703 = call "ips_switchHeaterOff.vi"("Instrument address"=w1351, "Rate"=w1350) -> ("B"=w1349:dbl)
                n704 = local write "Actual Field (T)"(w1349) -> ()
              }
            }
          }
        }
      }
      event "Go to Set": Value Change {
        n705 = event-data() -> ()  [unwired: 1 in, 6 out]
        n706 = local read "V/I (Ohm)"() -> (w1358:dbl)
        n707 = local read "B/V (T/V)"() -> (w1357:dbl)
        n708 = local read "Lock_in_Amplifier"() -> (w1354:refnum<visa-resource-name>)
        n709 = local read "Sweep Rate (T/min)"() -> (w1356:dbl)
        n710 = local read "Magnet"() -> (w1359:bool)
        n711 = call "Ramp_Field.vi"("Set Field (T) in"="Set Field (T)", "Sweep Rate (T/min)"=w1356, "V/I (Ohm)"=w1358, "error in (no error)"=w1360, "Magnet"=w1359, "B/V (T/V)"=w1357, "VISA Refnum in"=w1354) -> ("error out"=w1362:errorcluster, "Actual Voltage (V)"=w1352:dbl, "Set Field (T) out"=w1355:dbl)  [unwired: 2 in]
        n712 = local write "Actual B Field (T)"(w1355) -> ()
        n713 = local write "Actual Voltage (V)"(w1352) -> ()
      }
      event "Measure /Pause": Value Change {
        n714 = event-data() -> ("NewVal"=w1364:bool)  [unwired: 1 in, 5 out]
        n715 = local write "Measuring"(w1364) -> ()
      }
      event "Stop": Value Change {
        n716 = event-data() -> ()  [unwired: 1 in, 6 out]
        n717 = local read "Measuring"() -> (w1372:bool)
        n718 = case shown="True" w1372 {
          tunnel: w1371 -> [w1373 w1375]
          tunnel: [w1373 w1376] -> w1370
          frame False {
          }
          frame True {
            w1377 = FALSE ("Measuring")
            n719 = local read "Temp/Magnetic Field"() -> (w1374:bool)
            n720 = local read "SaveSweep"() -> (w1378:bool)
            n721 = local write "Measuring"(w1377) -> ()
            n722 = local write "Measure /Pause"(w1377) -> ()
            n723 = case shown="False" w1374 {
              tunnel: [w1382 w1391] -> w1376
              tunnel: w1375 -> [w1381 w1392]
              frame False {
                n724 = local read "Lock_in_Amplifier"() -> (w1383:refnum<visa-resource-name>)
                n725 = local read "V/I (Ohm)"() -> (w1387:dbl)
                n726 = local read "Sweep Rate (T/min)"() -> (w1386:dbl)
                n727 = local read "Set Field (T)"() -> (w1388:dbl)
                n728 = local read "B/V (T/V)"() -> (w1384:dbl)
                n729 = local read "Magnet"() -> (w1385:bool)
                n730 = call "Ramp_Field.vi"("Set Field (T) in"=w1388, "Sweep Rate (T/min)"=w1386, "V/I (Ohm)"=w1387, "error in (no error)"=w1381, "Magnet"=w1385, "B/V (T/V)"=w1384, "VISA Refnum in"=w1383) -> ("error out"=w1382:errorcluster, "Actual Voltage (V)"=w1379:dbl, "Set Field (T) out"=w1380:dbl)  [unwired: 2 in]
                n731 = local write "Actual B Field (T)"(w1380) -> ()
                n732 = local write "Actual Voltage (V)"(w1379) -> ()
              }
              frame True {
                n733 = local read "Set temperature (K)"() -> (w1389:dbl)
                n734 = Number To Fractional String(number=w1389, precision (6)=i16 3) -> (F-format string=w1395:string)  [unwired: 2 in]
                n735 = local read "Lake Shore"() -> (w1390:refnum<visa-resource-name>)
                n736 = Concatenate Strings("SETP 1," ("write buffer"), w1395) -> (w1393:string)
                n737 = VISA Write(VISA resource name=w1390, write buffer=w1393, error in (no error)=w1392) -> (error out=w1391:errorcluster)  [unwired: 2 out]
              }
            }
            n738 = case shown="True" w1378 {
              tunnel: w1374 -> [_ w1397]
              frame False {
              }
              frame True {
                w1404 = 1 ("index (row)")
                w1405 = 0 ("index (row)")
                n739 = case shown="True" w1397 {
                  tunnel: [w1421 w1423] -> w1415
                  tunnel: [w1420 w1422] -> w1398
                  frame True {
                    n740 = local read "Averaged P(T)"() -> (w1420:dbl[][])
                    n741 = local read "I(T) /Averaged/"() -> (w1421:cluster{"B array":dbl[], dbl[]}[])
                  }
                  frame False {
                    n742 = local read "Averaged P(B)"() -> (w1422:dbl[][])
                    n743 = local read "I(B) /Averaged/"() -> (w1423:cluster{"B array":dbl[], dbl[]}[])
                  }
                }
                n744 = local read "Measurement File_average"() -> (w1416:path)
                n745 = local read "Averaged dt"() -> (w1407:dbl[][])
                n746 = Index Array(array=w1407, index (row)=w1405) -> (element=w1406:dbl[])  [unwired: 1 in]
                n747 = Index Array(array=w1407, index (row)=w1404) -> (element=w1400:dbl[])  [unwired: 1 in]
                n748 = Index Array(array=w1415, index=1) -> (element=w1411:cluster{"B array":dbl[], dbl[]})
                n749 = Index Array(array=w1415, index=0) -> (element=w1412:cluster{"B array":dbl[], dbl[]})
                n750 = Unbundle(w1411) -> ("B array"=w1402:dbl[], w1401:dbl[])
                n751 = Unbundle(w1412) -> ("B array"=w1410:dbl[], w1409:dbl[])
                n752 = Index Array(array=w1398, index (row)=w1405) -> (element=w1403:dbl[])  [unwired: 1 in]
                n753 = Index Array(array=w1398, index (row)=w1404) -> (element=w1399:dbl[])  [unwired: 1 in]
                n754 = Build Array(w1410, w1409, w1406, w1403, w1402, w1401, w1400, w1399) -> (w1408:dbl[][])
                n755 = call-poly <vilib>:"Write Delimited Spreadsheet.vi"("file path (dialog if empty)"=w1416, "format (%.3f)"="%.5g", "2D data"=w1408, "append to file? (F)"=TRUE ("transpose? (F)"), "transpose? (F)"=TRUE ("append to file? (F)")) -> ()  [unwired: 9 in, 2 out]
              }
            }
          }
        }
      }
      event "Sweep": Value Change {
        n756 = event-data() -> ("NewVal"=w1427:bool)  [unwired: 1 in, 5 out]
        n757 = case shown="True" w1427 {
          frame False {
          }
          frame True {
            n758 = local read "Measurement File"() -> (w1428:path)
            n759 = Two Button Dialog(message="Do you want to create additional files for the sweeping measurements?" ("string"), 1:"No" ("F button name (\"Cancel\")"), 2:"Yes" ("T button name (\"OK\")")) -> (T button?=w1430:bool)
            n760 = case shown="True" w1430 {
              tunnel: w1428 -> [_ w1435]
              frame False {
                n761 = local write "SaveSweep"(FALSE ("SaveSweep")) -> ()
              }
              frame True {
                n762 = call "Create_sweep_files.vi"("Measurement File"=w1435) -> ("Path 3"=→"Measurement File_dn":path, "Path 2"=→"Measurement File_up":path, "Path"=→"Measurement File_average":path)  [unwired: 8 in]
                "SaveSweep" <- TRUE
              }
            }
          }
        }
      }
      event "Measure Noise": Value Change {
        n763 = event-data() -> ("NewVal"=w1442:bool)  [unwired: 1 in, 5 out]
        n764 = case shown="True" w1442 {
          frame False {
          }
          frame True {
            n765 = local read "Gain (V/A)"() -> (w1447:dbl)
            n766 = call "Noise_measurement.vi"("Gain (V/A)"=w1447, "Cycles"="Cycles", "Lower Cut-Off"="Cut-Off Frequency", "minimum value"="minimum value", "Filter On"="Filter On", "maximum value"="maximum value", "physical channels"="physical channels", "rate"="Rate", "samples per channel"="Samples per channel") -> ("Current (pA) Filtered"=→"Current (pA) Filtered":waveform(dbl), "PSD (pA/Hz^1/2) Peaks Removed"=→"PSD (pA/Hz^1/2) Peaks Removed":cluster{"f0":dbl, "df":dbl, "magnitude":dbl[]}, "Current (pA)"=→"Current (pA)":dbl[], "PSD (pA/Hz^1/2)"=→"PSD (pA/Hz^1/2)":cluster{"f0":dbl, "df":dbl, "magnitude":dbl[]})  [unwired: 3 in]
          }
        }
      }
      event "Calibrate": Value Change {
        n767 = event-data() -> ()  [unwired: 1 in, 6 out]
        n768 = case shown="True" "Calibrate" {
          frame False {
          }
          frame True {
            w1462 = dbl[] []
            n769 = while {
              shift-right: [w1495] -> w1460
              shift-left: dbl[][] [] -> [w1494]
              shift-right: [w1478] -> _
              shift-left: w1462 -> [w1490]
              shift-right: [w1487] -> _
              shift-left: w1462 -> [w1489]
              shift-right: [w1477] -> _
              shift-left: w1462 -> [w1488]
              shift-right: [w1469] -> _
              shift-left: 0.0 ("Set Field out") -> [w1468]
              stop <- w1491 stop-if-true
              n770 = call "Calibtarion.vi"("Dwell Time (ms)"="Dwell Time (ms)", "V array in (V)"=w1490, "I array in (A)"=w1488, "Collected array in"=w1494, "B array in (T)"=w1489, "Set Field (T)"=w1468, "dB"="dB") -> ("Best Linear Fit"=w1479:dbl[], "appended array"=→"appended array":dbl[][], "slope"=→"B/V (T/V)":dbl, "V array out (V)"=w1478:dbl[], "Boolean"=w1493:bool, "I array out (A)"=w1477:dbl[], "intercept 2"=→"I0 (A)":dbl, "Collected array out"=w1495:dbl[][], "intercept"=→"B0 (T)":dbl, "B array Out"=w1487:dbl[], "slope 2"=→"V/I (Ohm)":dbl, "Best Linear Fit 2"=w1484:dbl[], "Set Field out"=w1469:dbl)
              n771 = Bundle("I array out (A)"=w1477, "V array out (V)"=w1478) -> (w1486:T16)  [unwired: 1 in]
              n772 = Bundle("I array out (A)"=w1477, "Best Linear Fit"=w1479) -> (w1480:T17)  [unwired: 1 in]
              n773 = Bundle("V array out (V)"=w1478, "B array Out"=w1487) -> (w1482:T18)  [unwired: 1 in]
              n774 = Bundle("V array out (V)"=w1478, "Best Linear Fit 2"=w1484) -> (w1483:T19)  [unwired: 1 in]
              n775 = Or(x=w1493, y="stop 2") -> (x .or. y?=w1491:bool)
              n776 = Build Array(w1486, w1480) -> (→"V_I":T20)
              n777 = Build Array(w1482, w1483) -> (→"B_V":T21)
            }
            n778 = flat-sequence {
              tunnel: w1460 -> [w1466]
              frame #0 {
                n779 = Two Button Dialog(message="Do you want to save calibration file?") -> (T button?=w1465:bool)  [unwired: 2 in]
                n780 = case shown="True" w1465 {
                  tunnel: w1466 -> [_ w1467]
                  frame False {
                  }
                  frame True {
                    n781 = call-poly <vilib>:"Write Delimited Spreadsheet.vi"("2D data"=w1467) -> ()  [unwired: 13 in, 2 out]
                  }
                }
              }
            }
          }
        }
      }
      event "New Measurement File": Value Change {
        n782 = event-data() -> ()  [unwired: 1 in, 6 out]
        n783 = local read "Sweep"() -> (w1497:bool)
        n784 = Open/Create/Replace File(prompt="Please select measurement file\n", operation (0:open)=T5."replace or create with confirmation") -> (refnum out=w1503:refnum<file>)  [unwired: 4 in, 2 out]
        n785 = local write "refnum out"(w1503) -> ()
        n786 = Refnum to Path(1:w1503) -> (0:w1498:path)
        n787 = case shown="True" w1497 {
          tunnel: w1498 -> [_ w1506]
          frame False {
          }
          frame True {
            n788 = Two Button Dialog(message="Do you want to create additional files for the sweeping measurements?" ("string"), 1:"No" ("F button name (\"Cancel\")"), 2:"Yes" ("T button name (\"OK\")")) -> (T button?=w1508:bool)
            n789 = case shown="True" w1508 {
              tunnel: w1506 -> [_ w1516]
              frame False {
                n790 = local write "SaveSweep"(FALSE ("SaveSweep")) -> ()
              }
              frame True {
                n791 = call "Create_sweep_files.vi"("Measurement File"=w1516) -> ("Path 3"=w1513:path, "Path 2"=w1514:path, "Path"=w1515:path)  [unwired: 8 in]
                n792 = local write "Measurement File_dn"(w1513) -> ()
                n793 = local write "Measurement File_average"(w1515) -> ()
                n794 = local write "Measurement File_up"(w1514) -> ()
                n795 = local write "SaveSweep"(TRUE) -> ()
              }
            }
          }
        }
        n796 = local write "Measurement File"(w1498) -> ()
        n797 = local write "Offset?"(FALSE ("Offset?")) -> ()
        n798 = local write "First?"(TRUE ("First?")) -> ()
      }
      event "Heater On/Off": Value Change {
        n799 = event-data() -> ()  [unwired: 1 in, 6 out]
        n800 = case shown="False" "Heater On/Off" {
          tunnel: w1521 -> [w1526 w1532]
          tunnel: w1520 -> [w1524 w1533]
          tunnel: [w1523 w1531] -> w1519
          frame False {
            n801 = VISA Write(VISA resource name=w1526, write buffer="RANGE,1,0", error in (no error)=w1524) -> (error out=w1523:errorcluster)  [unwired: 2 out]
          }
          frame True {
            n802 = Number To Decimal String(number="Heater Range") -> (decimal integer string=w1529:string)  [unwired: 1 in]
            n803 = Concatenate Strings("RANGE,1," ("write buffer"), w1529) -> (w1527:string)
            n804 = VISA Write(VISA resource name=w1532, write buffer=w1527, error in (no error)=w1533) -> (error out=w1531:errorcluster)  [unwired: 2 out]
          }
        }
      }
      event "Set temperature (K)": Value Change {
        n805 = event-data() -> ()  [unwired: 1 in, 6 out]
        n806 = local read "Set temperature (K)"() -> (w1537:dbl)
        n807 = Number To Fractional String(number=w1537, precision (6)=i16 3) -> (F-format string=w1540:string)  [unwired: 2 in]
        n808 = Concatenate Strings("SETP 1," ("write buffer"), w1540) -> (w1538:string)
        n809 = VISA Write(VISA resource name=w1534, write buffer=w1538, error in (no error)=w1536) -> (error out=w1535:errorcluster)  [unwired: 2 out]
      }
      event "Temp Ramping Rate (K/min)": Value Change {
        n810 = event-data() -> ()  [unwired: 1 in, 6 out]
        n811 = local read "Temp Ramping Rate (K/min)"() -> (w1546:dbl)
        n812 = Number To Fractional String(number=w1546, precision (6)=i16 1) -> (F-format string=w1552:string)  [unwired: 2 in]
        n813 = Concatenate Strings("RAMP 1,1," ("string"), w1552) -> (w1551:string)
        n814 = VISA Write(VISA resource name=w1549, write buffer=w1551, error in (no error)=w1548) -> (error out=w1547:errorcluster)  [unwired: 2 out]
      }
      event "Heater Range": Value Change {
        n815 = event-data() -> ()  [unwired: 1 in, 6 out]
        n816 = local read "Heater On/Off"() -> (w1558:bool)
        n817 = case shown="True" w1558 {
          tunnel: w1557 -> [w1559 w1564]
          tunnel: [w1559 w1563] -> w1556
          tunnel: w1554 -> [_ w1562]
          frame False {
          }
          frame True {
            n818 = local read "Heater Range"() -> (w1560:enum16{"Off", "Low", "Medium", "High"})
            n819 = Number To Decimal String(number=w1560) -> (decimal integer string=w1566:string)  [unwired: 1 in]
            n820 = Concatenate Strings("RANGE,1," ("write buffer"), w1566) -> (w1565:string)
            n821 = VISA Write(VISA resource name=w1562, write buffer=w1565, error in (no error)=w1564) -> (error out=w1563:errorcluster)  [unwired: 2 out]
          }
        }
      }
    }
    n822 = Reciprocal(x="Sampling rate (Hz)") -> (1/x=w1185:dbl)
    n823 = Multiply(x=w1185, y=1000.0) -> (x*y=w1183:dbl)
    n824 = Wait Until Next ms Multiple(millisecond multiple=w1183) -> ()  [unwired: 1 out]
  }
  n825 = local read "Field Step (T)"() -> (w6:dbl)
  n826 = local read "Max Field (T)"() -> (w89:dbl)
  n827 = local read "dB (T)"() -> (w7:dbl)
  n828 = local read "Min Field (T)"() -> (w90:dbl)
  n829 = Select(t=w6, s=w4, f=w7) -> (s? t:f=w5:dbl)
  n830 = Divide(x=w89, y=w5) -> (x/y=w91:dbl)
  n831 = for {
    N: w91 -> [_]
    tunnel: w5 -> [w1571]
    tunnel: [w1568] -> w52 mode=indexing
    tunnel: w90 -> [w1569]
    tunnel: [0.0] -> _ mode=indexing
    i -> [w1572]
    n832 = Multiply(x=w1572, y=w1571) -> (x*y=w1570:dbl)
    n833 = Add(x=w1570, y=w1569) -> (x+y=w1568:dbl)
  }
  n834 = Multiply(x=w52, y=0.0) -> (x*y=w49:dbl[])
  n835 = Array Size(array=w49) -> (size(s)=w48:i32)
  n836 = Decrement(x=w48) -> (x-1=w47:i32)
  n837 = local write "B array"(w52) -> ()
  n838 = Array Subset(array=w49, length=w47) -> (w46:dbl[])  [unwired: 1 in]
  n839 = Build Array(w49, w49) -> (w50:dbl[][])
  n840 = local read "Max temperature (K)"() -> (w19:dbl)
  n841 = local read "Min Temperature (K)"() -> (w21:dbl)
  n842 = local write "Averaged I(B)"(w50) -> ()
  n843 = Build Array(w46, w46) -> (w45:dbl[][])
  n844 = Divide(x=w19, y="dt (K)") -> (x/y=w22:dbl)
  n845 = local write "Averaged P(B)"(w45) -> ()
  n846 = local write "Averaged dt"(w45) -> ()
  n847 = for {
    N: w22 -> [_]
    tunnel: "dt (K)" -> [w1577]
    tunnel: [w1574] -> w11 mode=indexing
    tunnel: w21 -> [w1575]
    tunnel: [0.0] -> _ mode=indexing
    i -> [w1578]
    n848 = Multiply(x=w1578, y=w1577) -> (x*y=w1576:dbl)
    n849 = Add(x=w1576, y=w1575) -> (x+y=w1574:dbl)
  }
  "T array" <- w11
  n850 = Multiply(x=w11, y=0.0) -> (x*y=w10:dbl[])
  n851 = Array Size(array=w10) -> (size(s)=w14:i32)
  n852 = Decrement(x=w14) -> (x-1=w15:i32)
  n853 = Array Subset(array=w10, length=w15) -> (w16:dbl[])  [unwired: 1 in]
  n854 = Build Array(w10, w10) -> (w13:dbl[][])
  n855 = local write "Averaged I(T)"(w13) -> ()
  n856 = Build Array(w16, w16) -> (w17:dbl[][])
  n857 = local write "Averaged P(T)"(w17) -> ()
  n858 = local write "Averaged dt"(w17) -> ()
  n859 = local read "Lake Shore"() -> (w100:refnum<visa-resource-name>)
  n860 = local read "IV converter"() -> (w116:refnum<visa-resource-name>)
  n861 = local read "Magnetic Field"() -> (w115:refnum<visa-resource-name>)
  n862 = VISA Close(VISA resource name=w116, error in (no error)=w118) -> (error out=w119:errorcluster)
  n863 = VISA Close(VISA resource name=w115, error in (no error)=w119) -> (error out=w117:errorcluster)
  n864 = Release Queue(queue=w123, error in (no error)=w117) -> (error out=w113:errorcluster)  [unwired: 1 in, 2 out]
  n865 = Merge Errors(w113, w112) -> (w114:errorcluster)
  n866 = VISA Close(VISA resource name=w100, error in (no error)=w114) -> (error out=w111:errorcluster)
  n867 = local read "refnum out"() -> (w109:refnum<file>)
  n868 = Close File(refnum=w109, error in=w111) -> (error out=w110:errorcluster)  [unwired: 1 out]
  n869 = call <vilib>:"Simple Error Handler.vi"("error in (no error)"=w110) -> ()  [unwired: 4 in, 5 out]
  "i" <- w82
  "j" <- w82
